vi "FisHRateZ-Main.vi"() -> ()   [LabVIEW 2014]
uses:
  ND2_Reader_32bit/controls/cluster_LIMLOCALMETADATA.ctl
  QSM/Queue_TESTGUIUPDATE/Controls/TypeDef_FrontPanelReferences.ctl
  QSM/Queue_TEST/Controls/QSM_RunStates.ctl
  QSM/Queue_TESTGUIUPDATE/Controls/QSM_RunStates.ctl
  Custom Controls/cluster - Image Results.ctl
  Utilities/Global - Demo Mode Flags.vi
  ND2_Reader_32bit/ND2_Reader_32.lvlib
  QSM/Queue_TESTGUIUPDATE/GUIUpdateQSM.lvlib
  QSM/QueueMaintenance/QueueMaintenance.lvlib
  QSM/Queue_TEST/TestQSM.lvlib
panel:
  in  "About":bool
  in  "Show ROI Detection GUI":bool
  in  "Directory ROI Processing":bool
  in  "Directory Complete Processing":bool
  in  "System Parameters":bool
  in  "Single ROI Calc":bool
  in  "Single File Processing":bool
  in  "Exit":bool
  out "ROI Found?":bool
  in  "Stop Processing":bool
  out "Status":string
  in  "Tab Control":T1(tab)
  in  "Original Image Zoom to Fit":bool
  in  "ROI FOUND Zoom to Fit":bool
  out "LIMLOCALMETADATA":T2 {"dTimeMSec" format="%.2f"}
  out "ROIS":dbl[](array[numeric]) format="%#.2g"
  out "Original Image":T3(plugin-control)
  out "ROI Found":T3(plugin-control)
  out "File":string
  out "XY Graph":cluster{"X":dbl[], "Y":dbl[]}[](graph)
  out "Results String":string
  out "Image Copy":T3(plugin-control)
  in  "Copy Zoom to Fit Image":bool
  in  "Save ROI Results":bool
  out "ROI Results":T4(array[cluster]) {"ROI Values" format="%#.2g"}
  # "* Note: Processing will go faster if 'Original Image' Tab is hidden"
  # "File"
  # "ROI FOUND?"
  # "ROI Values of First Frame"
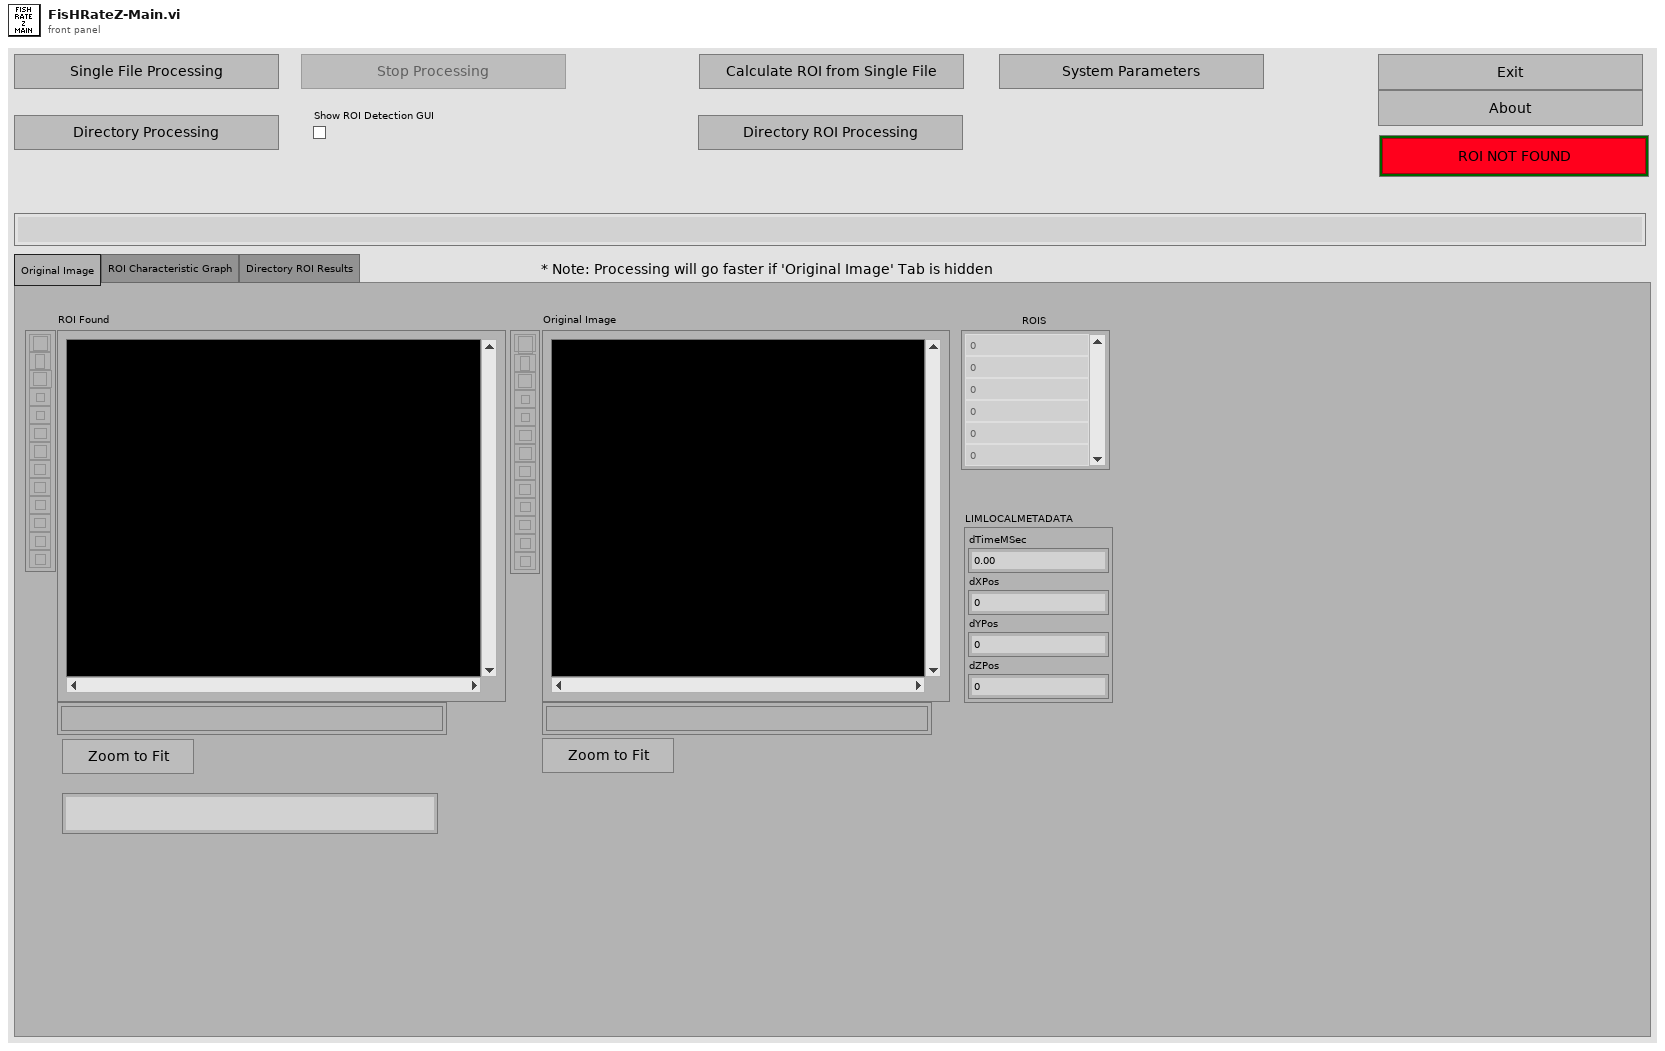
[diagram p1: front panel]
types:
  T1 = enum32{"Original Image", "ROI Characteristic Graph", "Directory ROI Results"}
  T2 = typedef "cluster_LIMLOCALMETADATA.ctl" = cluster{"dTimeMSec":dbl, "dXPos":dbl, "dYPos":dbl, "dZPos":dbl}
  T3 = typedef "IMAQ Image.ctl" = refnum<image>
  T4 = cluster{"File":string, "ROI Found?":bool, "ROI Values":dbl[]}[]
  T5 = typedef "GUIUpdateQSM.lvlib/TypeDef_FrontPanelReferences.ctl" = cluster{"Start":refnum<vi>, "Stop":refnum<vi>, "Status":refnum<vi>, "Exit Button":refnum<vi>, "This VI":refnum<vi>, "System Parameters":refnum<vi>, "Single ROI Calc":refnum<vi>, "ROI X-Y Graph":refnum<vi>, "Directory Complete Processing":refnum<vi>, "Directory ROI Processing":refnum<vi>}
  T6 = typedef "QueueMaintenance.lvlib/QSMRef_ALL.ctl" = cluster{"QSMRef_UpdateUI":T7, "QSMRef_TEST":T8}
  T7 = typedef "GUIUpdateQSM.lvlib/QSM_Reference.ctl" = refnum<queue>
  T8 = typedef "TestQSM.lvlib/QSM_Reference.ctl" = refnum<queue>
  T9 = typedef "TestQSM.lvlib/QSM_ShiftRegister.ctl" = cluster{"Queue References":T6, "user event in":refnum<user-event>, "Single File to Process":path, "Single Image Results":T10, "Analysis Start":timestamp, "Directory to Process":path, "Index":i32, "All Files to Process":path[], "ROI Process":cluster{"Any ROI FOUND?":bool, "ROIS":T11[], "ROIS Found?":bool[], "Particle Measurements (Pixels)":dbl[][], "Particle Variables":i32[], "N Particles Found":i32, "N ROIS Found":i32, "Circles for each Particle":cluster{"Pos. X":i32, "Pos. Y":i32, "Radius":i32, "Core Area":i32}[]}}
  T10 = typedef "cluster - Image Results.ctl" = cluster{"Filename":path, "ROI Results":cluster{"ROIS":dbl[], "LIMLOCALMETADATA":T2}[], "User Stopped?":bool, "ROI Found?":bool, "Error":errorcluster}
  T11 = typedef "ROI Descriptor" = cluster{"Global Rectangle":i32[], "Contours":cluster{"ID":enum32{"External", "Internal"}, "Type":u32, "Coordinates":i32[]}[]}
  T12 = typedef "TestQSM.lvlib/QSM_RunStates.ctl" = enum16{"NULL", "Sect01-Initialize-00-GROUP.ENQUEUE", "Sect02-Single File_Check for Parameters", "Sect02-Single File_Ask for File", "Sect02-Single File_Run Analysis", "Sect02-Single File_Write Results", "Sect03-Single ROI Calc_Check for Parameters", "Sect03-Single ROI Calc_Ask for File", "Sect03-Single ROI Calc_Run Analysis", "Sect03-Single ROI _Write Results", "Sect12-Full Dir_Check for Parameters", "Sect12-Full Dir_Ask for Dir", "Sect12-Full Dir_Check for Next Image to Process", "Sect12-Full Dir_Run Analysis", "Sect12-Full Dir_Write Results", "Sect12-Full Dir_Check if User Stopped", "Sect13-FullDir ROI Calc_Check for Parameters", "Sect13-FullDir ROI Calc_Ask for Dir", "Sect13-Full Dir ROI Calc_Check for Next Image to Process", "Sect13-Full Dir ROI Calc_Run Analysis", "Sect13-Full Dir ROI Calc_Write Results", "Sect13-Full Dir ROI Calc_Check if User Stopped", "Sect90-GUI_Config_Change UI Before Analysis", "Sect90-GUI_Config_Change UI After Analysis", "Sect90-GUI_Stop Processing Pressed", "Sect90-GUI_Stop Processing Button Set Back to F", "Sect90-GUI_Clear ROIs", "Sect99_EXIT-00-Group.Enqueue", "Sect99_EXIT-01-StopQSM"}
  T13 = cluster{"File":string, "ROI Found? 2":bool, "ROIS 2":dbl[]}[]
  T14 = typedef "GUIUpdateQSM.lvlib/QSM_RunStates.ctl" = enum16{"NULL", "Sect01_Initialize-00_GROUP.ENQUEUE", "Sect01_Initialize-01_SetMainToDefault", "Sect01_Initialize-02_Clear Status Strings", "Sect02_UpdateUI-00_Enable Stop_ Disable Start", "Sect02_UpdateUI-01_Enable Start_Disable Stop", "Sect02_UpdateUI-02_Update Status String", "Sect02_UpdateUI-03_Clear XY-Graph", "Sect03-Open ROI  GUI", "Sect03-Close ROI GUI", "Sect99_EXIT-00_Group.Enqueue", "Sect99_EXIT-01_CloseReferences", "Sect99_EXIT-02_StopQSM"}
  T15 = typedef "cluster_LIMPICTURE.ctl" = cluster{"uiWidth":u32, "uiHeight":u32, "uiBitsPerComp":u32, "uiComponents":u32, "uiWidthBytes":u32, "uiSize":u32, "pImageData":u32}
  T16 = typedef "numeric_LIMFILEHANDLE.ctl" = i32
  T17 = cluster{"ROI Calculation":dbl[], "LIMLOCALMETADATA":T2}
  T18 = cluster{"Global Rectangle":i32[], "Contours":cluster{"Contour Type":u32, "ROI Type":u32, "Points":i32[]}[]}
  T19 = cluster{"name":string, "ROI Found?":bool, "ROIS":dbl[]}
  T20 = cluster{"name":string, "ROI Found?":bool, "ROIS":dbl[]}[]
  T21 = typedef "Image Type" = u32
  T22 = cluster{"ROI Calculation":dbl[], "LIMLOCALMETADATA":T2}[]
  T23 = typedef "GUIUpdateQSM.lvlib/QSM_ShiftRegister.ctl" = cluster{"Queue References":T6, "GUI(i) Refs":T5, "user event in":refnum<user-event>}
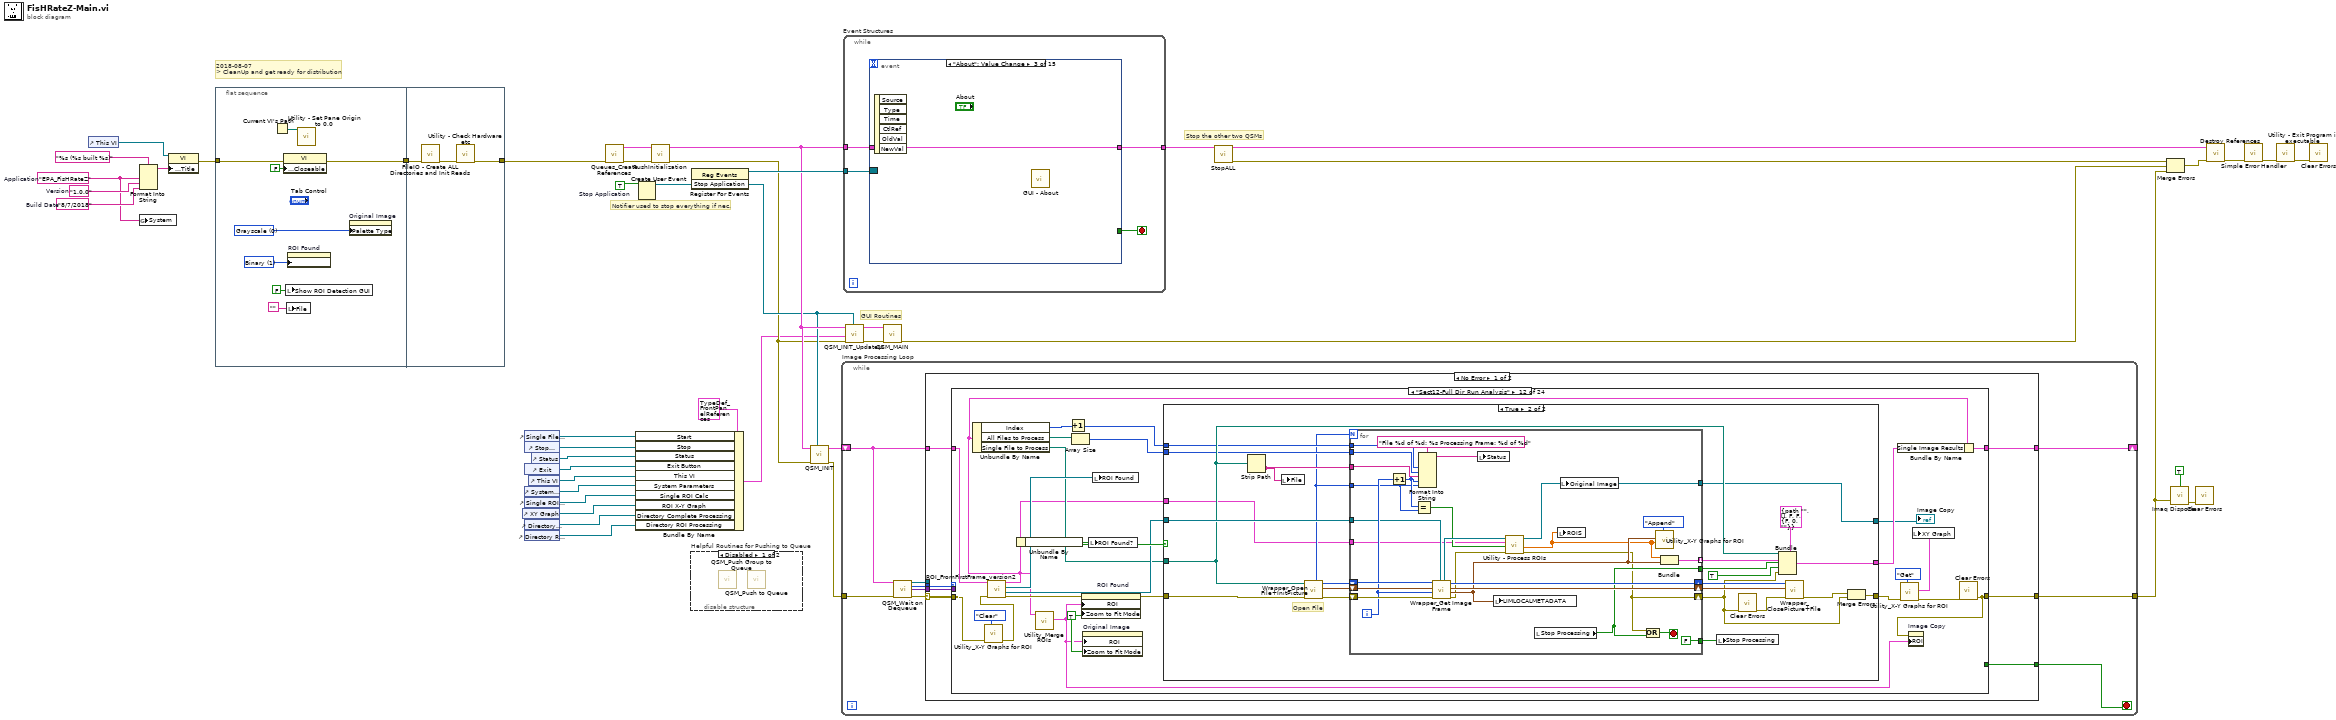
[diagram p0: block diagram]
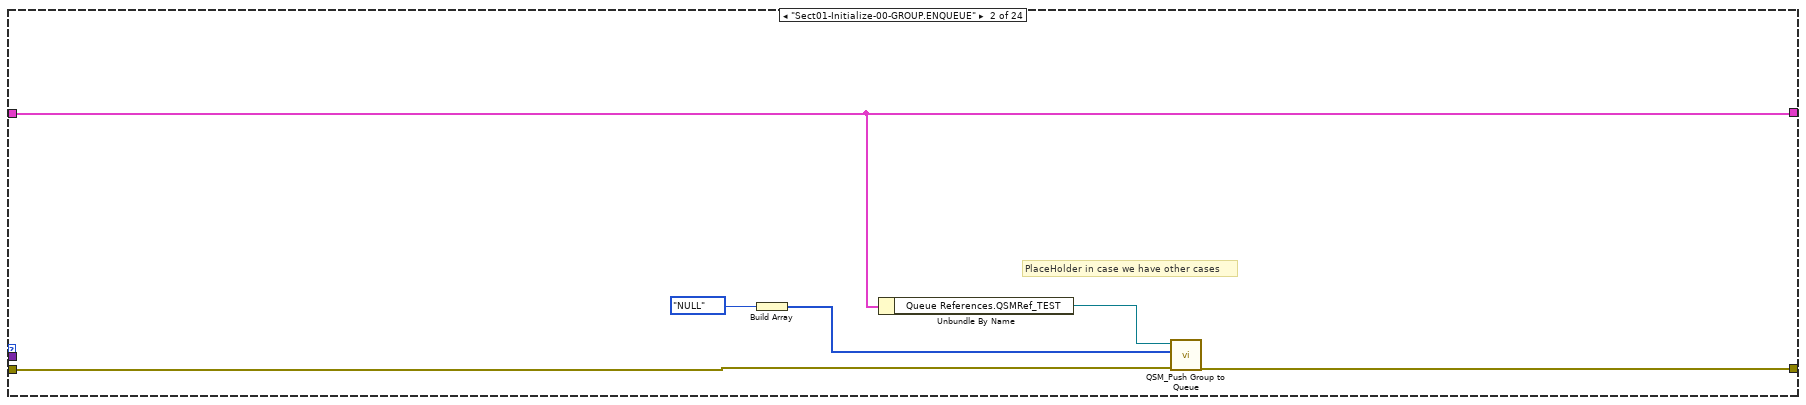
[diagram p4: hidden frame]
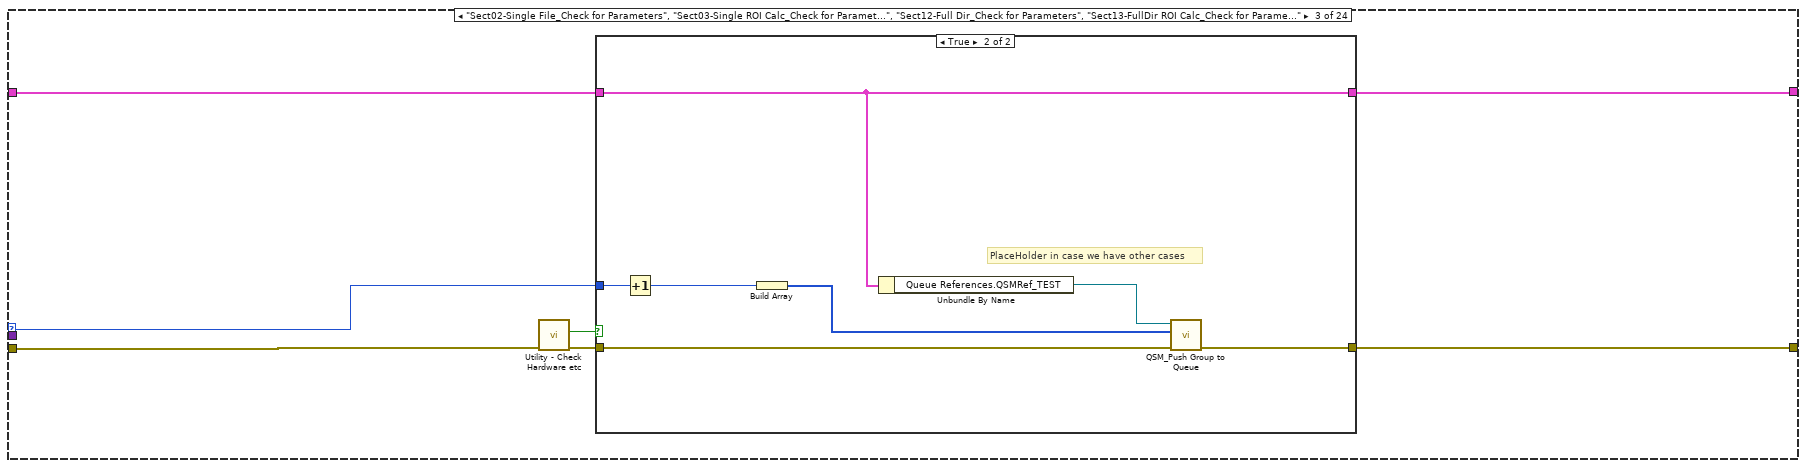
[diagram p5: hidden frame]
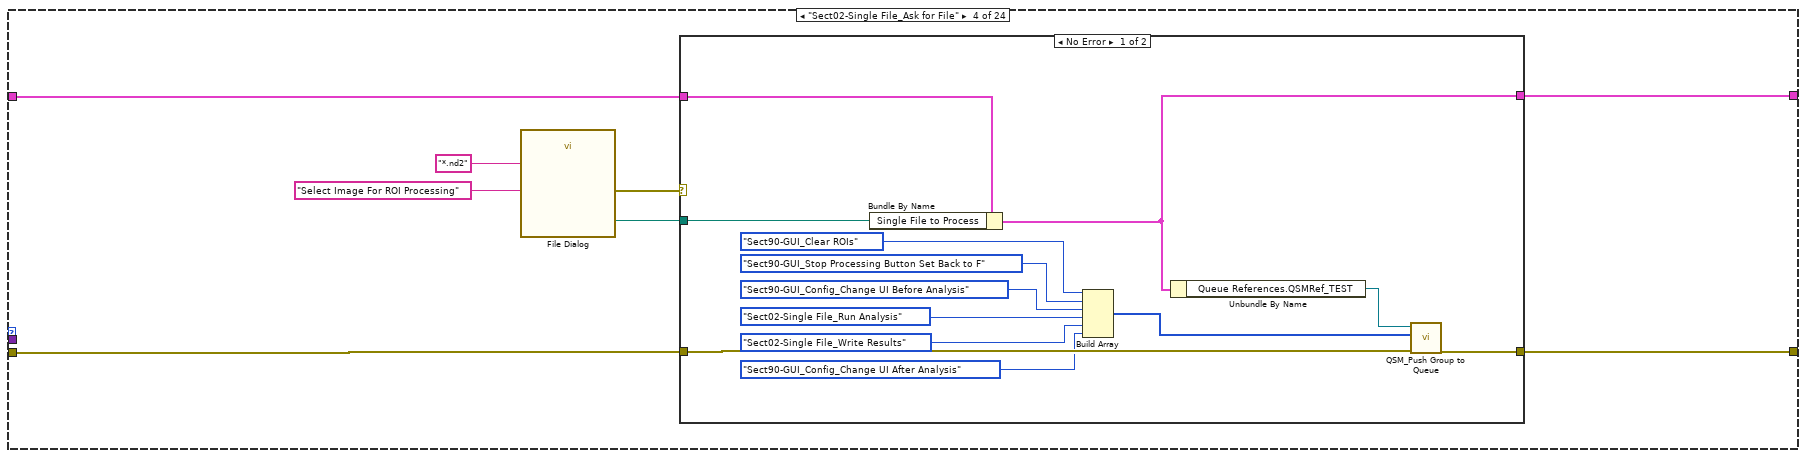
[diagram p7: hidden frame]
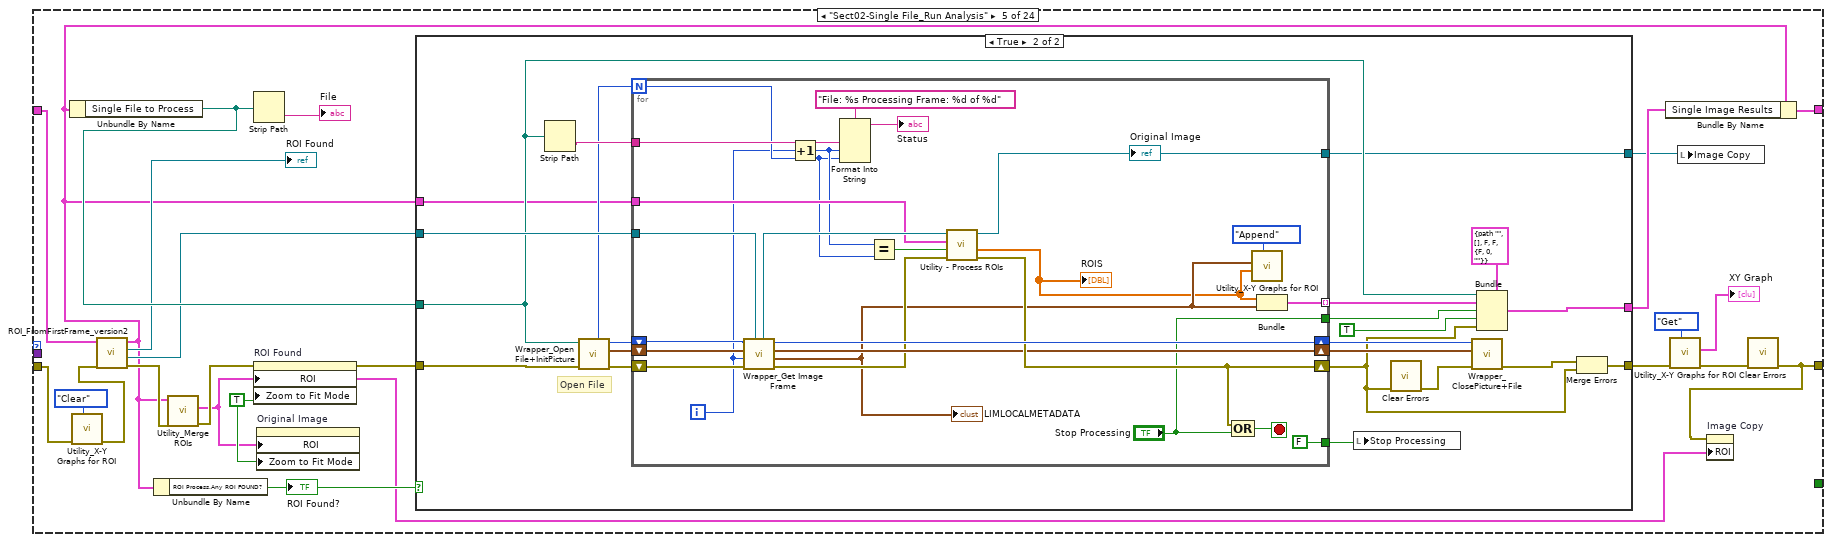
[diagram p9: hidden frame]
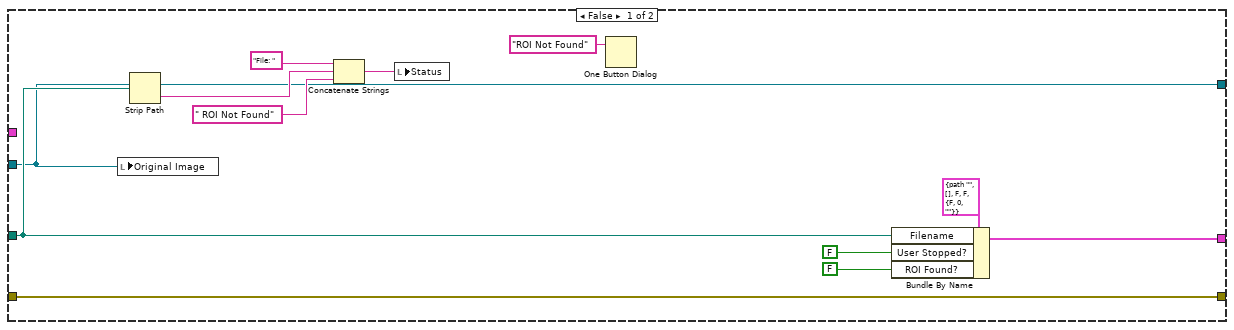
[diagram p10: hidden frame]
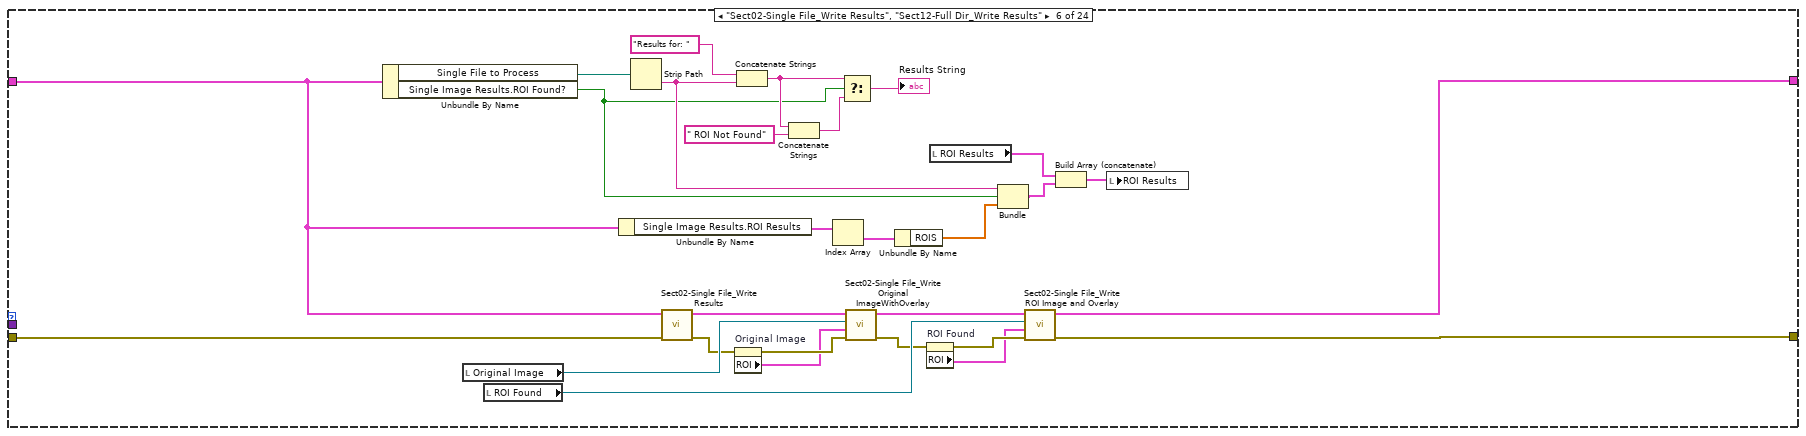
[diagram p11: hidden frame]
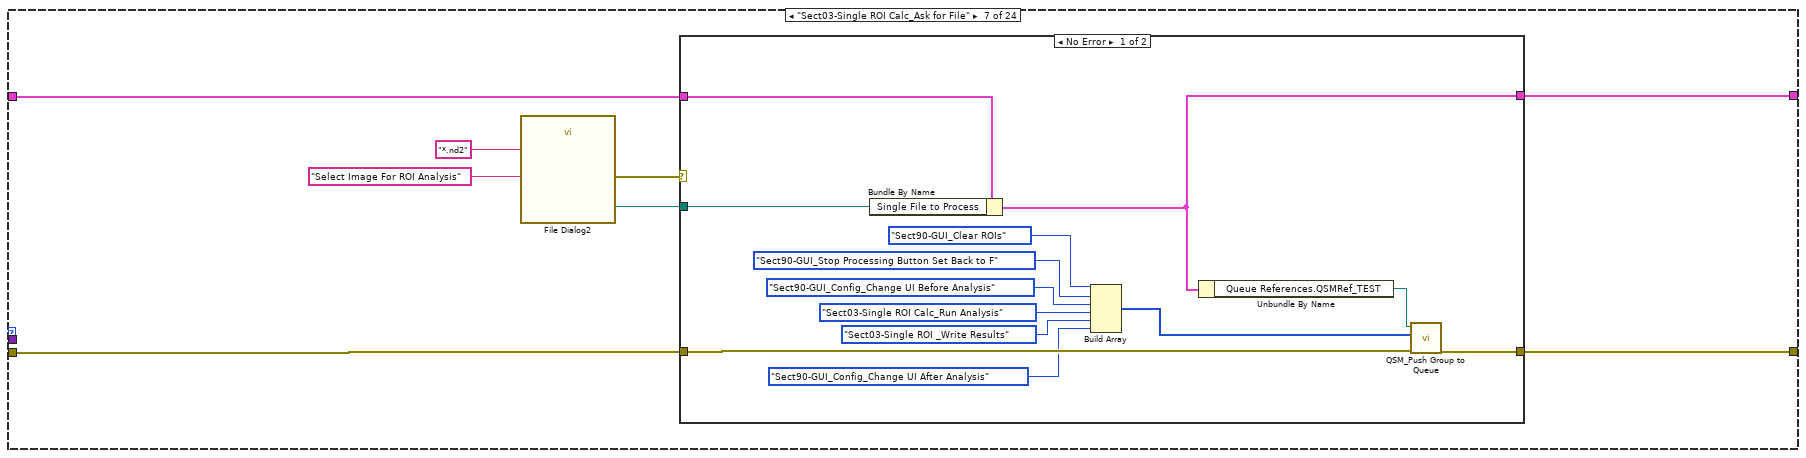
[diagram p12: hidden frame]
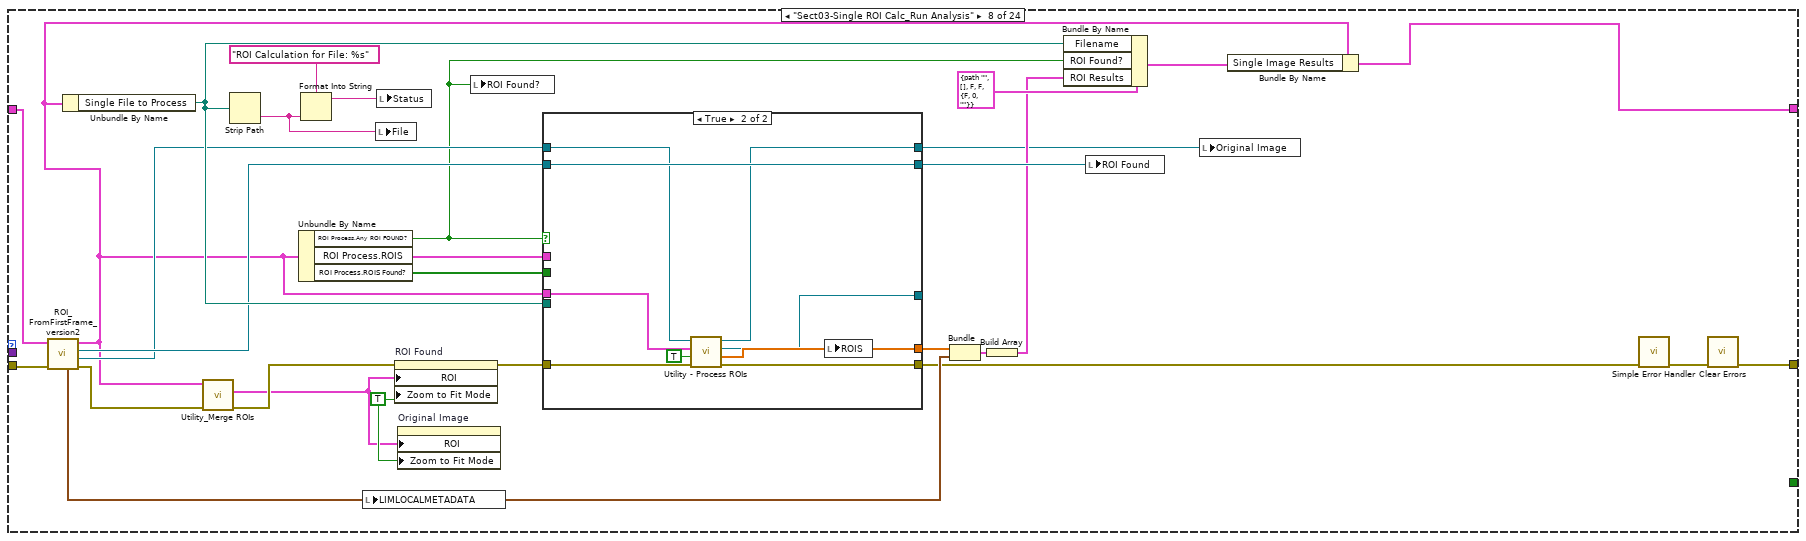
[diagram p14: hidden frame]
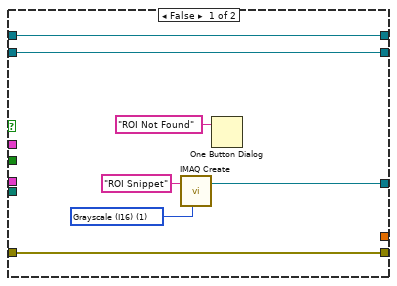
[diagram p15: hidden frame]
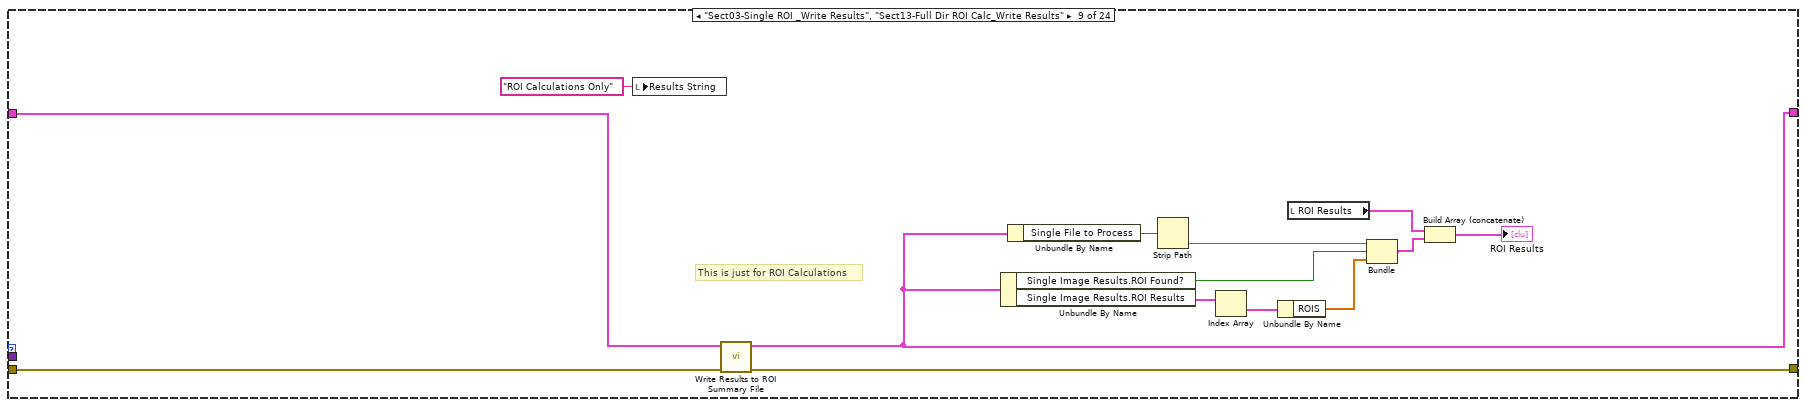
[diagram p16: hidden frame]
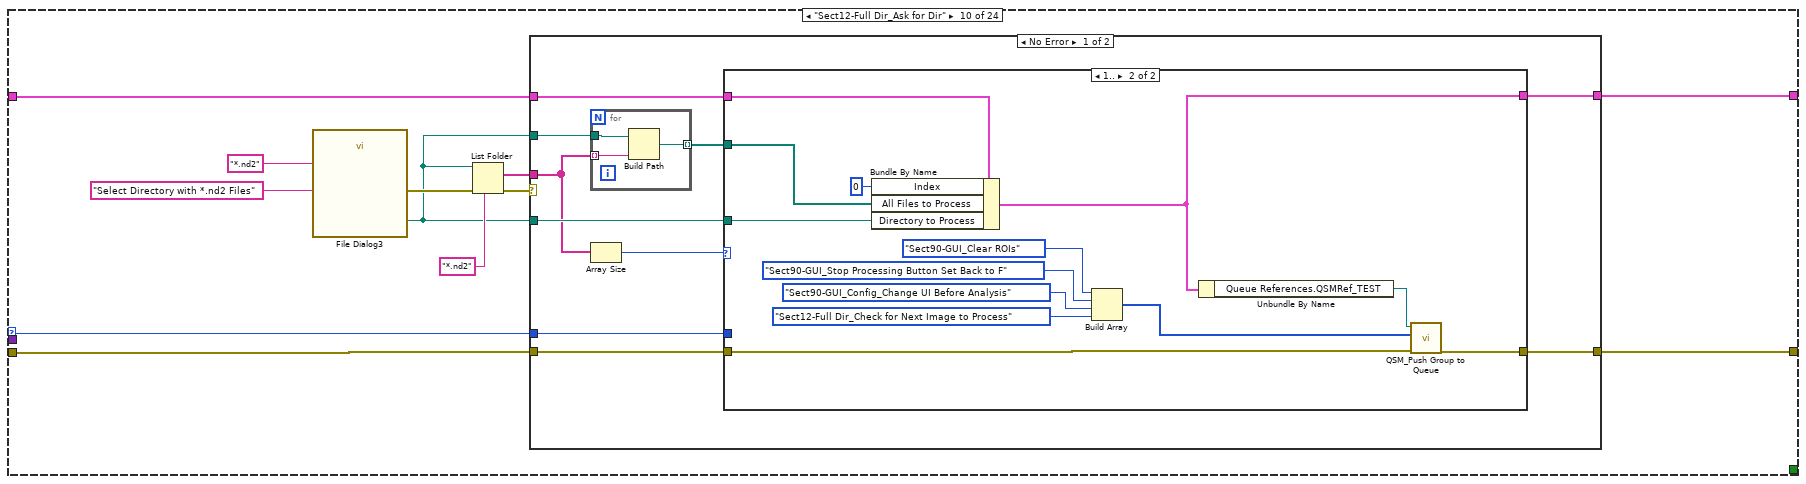
[diagram p17: hidden frame]
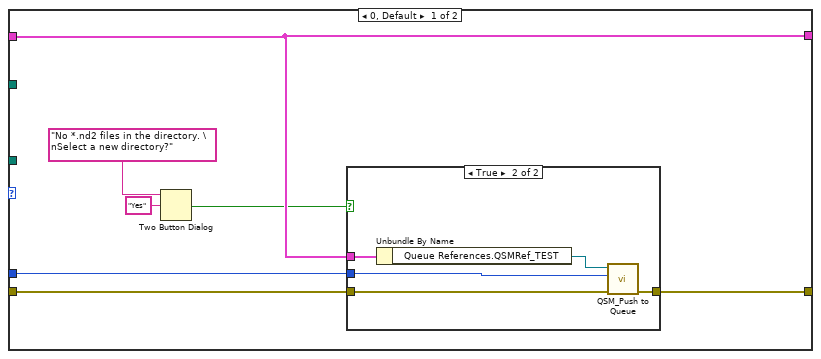
[diagram p18: hidden frame]
diagram:
  w31 = TRUE  # Stop Application
  w42 = "8/7/2018"  # Build Date
  w38 = "EPA_FisHRateZ"  # Application
  w43 = "1.0.0"  # Version
  # "GUI Routines"
  # "Stop the other two QSMs"
  # "2018-08-07\n> CleanUp and get ready for distribution"
  # "Notifier used to stop everything if nec."
  n1 = control-ref of="This VI"() -> (w39:refnum<vi>)
  n2 = Format Into String(format string="%s (%s built %s)", w38, w43, w42) -> (resulting string=w40:string)  [unwired: 2 in, 1 out]
  n3 = global write "Global - Demo Mode Flags.vi" "System"(w38) -> ()
  n4 = property class="VI"(reference=w39, "Front Panel.Title"=w40) -> (error out=w37:errorcluster)  [unwired: 1 in, 1 out]
  n5 = flat-sequence {
    tunnel: w37 -> [w50]
    tunnel: [w46] -> w13
    tunnel: w13 -> [w54]
    tunnel: [w52] -> w12
    frame #0 {
      w49 = u32 1 items=["Grayscale", "Binary", "Gradient", "Rainbow", "Temperature", "User Defined"] ("Palette")
      w48 = u32 0 items=["Grayscale", "Binary", "Gradient", "Rainbow", "Temperature", "User Defined"] ("Palette")
      n6 = Current VI's Path() -> (path=w47:path)
      n7 = property class="VI"(error in=w50, "Front Panel.Closeable"=FALSE ("Front Panel Window:Closeable")) -> (error out=w46:errorcluster)  [unwired: 1 in, 1 out]
      n8 = local write "Show ROI Detection GUI"(FALSE ("Show ROI Detection GUI")) -> ()
      n9 = local write "File"("") -> ()
      n10 = property on="ROI Found" class="ImageControl"("Palette:Palette Type"=w49) -> ()  [unwired: 2 in, 2 out]
      n11 = call "Utility - Set Pane Origin to 0,0.vi"("vi path"=w47) -> ()  [unwired: 10 in, 1 out]
      n12 = property on="Original Image" class="ImageControl"("Palette Type"=w48) -> ()  [unwired: 2 in, 2 out]
    }
    frame #1 {
      n13 = call "FileIO - Create ALL Directories and Init Reads.vi"("error in"=w54) -> ("error out"=w53:errorcluster)  [unwired: 9 in]
      n14 = call "Utility - Check Hardware etc.vi"("error in"=w53) -> ("error out"=w52:errorcluster)  [unwired: 8 in, 1 out]
    }
  }
  n15 = control-ref of="XY Graph"() -> (w8:refnum<vi>)
  n16 = control-ref of="Single File Processing"() -> (w19:refnum<vi>)
  n17 = control-ref of="Stop Processing"() -> (w20:refnum<vi>)
  n18 = control-ref of="Exit"() -> (w17:refnum<vi>)
  n19 = control-ref of="System Parameters"() -> (w15:refnum<vi>)
  n20 = control-ref of="Single ROI Calc"() -> (w9:refnum<vi>)
  n21 = control-ref of="Directory Complete Processing"() -> (w7:refnum<vi>)
  n22 = control-ref of="Directory ROI Processing"() -> (w6:refnum<vi>)
  n23 = control-ref of="This VI"() -> (w16:refnum<vi>)
  n24 = control-ref of="Status"() -> (w18:refnum<vi>)
  n25 = call "Queues_Create References.vi"("error in"=w12) -> ("error out"=w32:errorcluster, "Queue References"=w33:T6)  [unwired: 8 in]
  n26 = Bundle By Name(cluster=T5 {"Start"=refnum, "Stop"=refnum, "Status"=refnum, "Exit Button"=refnum, "This VI"=refnum, "System Parameters"=refnum, "Single ROI Calc"=refnum, "ROI X-Y Graph"=refnum, "Directory Complete Processing"=refnum, "Directory ROI Processing"=refnum} ("FP References"), "Start"=w19, "Stop"=w20, "Status"=w18, "Exit Button"=w17, "This VI"=w16, "System Parameters"=w15, "Single ROI Calc"=w9, "ROI X-Y Graph"=w8, "Directory Complete Processing"=w7, "Directory ROI Processing"=w6) -> (w5:T5)
  n27 = Create User Event(user event datatype=w31) -> (user event=w24:refnum<user-event>)  [unwired: 1 in, 1 out]
  n28 = call "PushInitialization.vi"("error in (no error)"=w32, "Queue References"=w33) -> ("error out"=w10:errorcluster, "Queue References"=w29:T6)  [unwired: 8 in]
  n29 = disable-structure "Helpful Routines for Pushing to Queue" shown="Disabled" {
    frame Disabled {
      n30 = call "QSM_Push Group to Queue.vi"() -> ()  [unwired: 11 in, 1 out]
      n31 = call "QSM_Push to Queue.vi"() -> ()  [unwired: 10 in, 2 out]
    }
    frame Enabled {
    }
  }
  n32 = register-events(w24) -> (reference out=w30:refnum<event-registration>)  [unwired: 2 in, 1 out]
  n33 = call "QSM_INIT.vi"("user event in"=w24, "error in"=w10, "Queue References"=w29) -> ("error out"=w23:errorcluster, "QSM_ShiftRegister_TEST"=w25:T9)  [unwired: 7 in]
  n34 = while "Image Processing Loop" {
    tunnel: [w57] -> w2
    shift-right: [w56] -> _
    shift-left: w25 -> [w63]
    tunnel: w23 -> [w62]
    stop <- w55 stop-if-true
    n35 = call "QSM_Wait on Dequeue.vi"("QSM_ShiftRegister in"=w63, "error in (no error)"=w62) -> ("Queue References.QSMRef out"=w61:T8, "RunStates_TEST"=w59:T12, "DATA.VARIANT"=w58:variant, "error out"=w60:errorcluster)  [unwired: 9 in, 1 out]
    n36 = case shown="No Error" w60 {
      selector: w60 -> [w64 w687]
      tunnel: [w70 w690] -> w57
      tunnel: w63 -> [w67 w689]
      tunnel: w61 -> [_ _]
      tunnel: w59 -> [w69 _]
      tunnel: w58 -> [w68 _]
      tunnel: [w66 w689] -> w56
      tunnel: [w65 TRUE] -> w55
      frame No Error {
        n37 = case shown="\"Sect12-Full Dir_Run Analysis\"" w69 {
          selector: w69 -> [_ _ w79 _ _ _ _ _ _ w310 w371 _ w483 w502 w563 _ w625 _ _ _ _ _ _ _]
          tunnel: w64 -> [w72 w76 w85 w101 w136 w227 w234 w267 w297 w315 w372 w404 w484 w507 w564 w609 w626 w652 w664 w669 w671 w676 w681 w684]
          tunnel: [w72 w75 w84 w100 w118 w216 w233 w277 w296 w320 w374 w392 w486 w512 w566 w604 w628 w651 w656 w665 w671 w676 w680 w684] -> w70
          tunnel: w68 -> [_ _ _ _ _ _ _ _ _ _ _ _ _ _ _ _ _ _ _ _ _ _ _ _]
          tunnel: w67 -> [w71 w78 w82 w102 w130 w200 w235 w262 w298 w321 w370 w400 w482 w513 w562 w588 w624 w655 w663 w668 w672 w677 w683 w686]
          tunnel: [w71 w78 w81 w96 w140 w217 w229 w274 w299 w317 w373 w416 w485 w509 w565 w601 w627 w654 w663 w668 w672 w677 w683 w686] -> w66
          tunnel: [_ _ _ _ _ _ _ _ _ _ _ _ _ _ _ _ _ _ _ _ _ _ _ TRUE] -> w65
          frame "NULL" {
          }
          frame "Sect01-Initialize-00-GROUP.ENQUEUE" {
            # "PlaceHolder in case we have other cases"
            n38 = Build Array(QSM_RunStates."NULL" ("QSM_RunStates_TEST")) -> (w73:T12[])
            n39 = Unbundle By Name(w78) -> ("Queue References.QSMRef_TEST"=w77:T8)
            n40 = call "QSM_Push Group to Queue.vi"("error in (no error)"=w76, "Group Cmds to Push"=w73, "QSM_Reference"=w77) -> ("error out"=w75:errorcluster)  [unwired: 8 in]
          }
          frame "Sect02-Single File_Check for Parameters", "Sect03-Single ROI Calc_Check for Parameters", "Sect12-Full Dir_Check for Parameters", "Sect13-FullDir ROI Calc_Check for Parameters" {
            n41 = call "Utility - Check Hardware etc.vi"("error in"=w85) -> ("error out"=w83:errorcluster, "OK?"=w80:bool)  [unwired: 8 in]
            n42 = case shown="True" w80 {
              tunnel: w82 -> [w87 w90]
              tunnel: [w86 w92] -> w84
              tunnel: w83 -> [w86 w91]
              tunnel: [w87 w90] -> w81
              tunnel: w79 -> [_ w89]
              frame False {
              }
              frame True {
                # "PlaceHolder in case we have other cases"
                n43 = Increment(x=w89) -> (x+1=w88:T12)
                n44 = Build Array(w88) -> (w93:T12[])
                n45 = Unbundle By Name(w90) -> ("Queue References.QSMRef_TEST"=w94:T8)
                n46 = call "QSM_Push Group to Queue.vi"("error in (no error)"=w91, "Group Cmds to Push"=w93, "QSM_Reference"=w94) -> ("error out"=w92:errorcluster)  [unwired: 8 in]
              }
            }
          }
          frame "Sect02-Single File_Ask for File" {
            n47 = call "File Dialog"("prompt"="Select Image For ROI Processing", "pattern (all files)"="*.nd2") -> ("selected path"=w95:path, "error out"=w97:errorcluster)  [unwired: 10 in, 2 out]
            n48 = case shown="No Error" w97 {
              tunnel: w102 -> [w109 w117]
              tunnel: w101 -> [w114 w116]
              tunnel: [w113 w116] -> w100
              tunnel: [w108 w117] -> w96
              tunnel: w95 -> [w110 _]
              frame No Error {
                n49 = Bundle By Name(cluster=w109, "Single File to Process"=w110) -> (w108:T9)
                n50 = Build Array(QSM_RunStates."Sect90-GUI_Clear ROIs" ("QSM_RunStates_TEST"), QSM_RunStates."Sect90-GUI_Stop Processing Button Set Back to F" ("QSM_RunStates_TEST"), QSM_RunStates."Sect90-GUI_Config_Change UI Before Analysis" ("QSM_RunStates_TEST"), QSM_RunStates."Sect02-Single File_Run Analysis" ("QSM_RunStates_TEST"), QSM_RunStates."Sect02-Single File_Write Results" ("QSM_RunStates_TEST"), QSM_RunStates."Sect90-GUI_Config_Change UI After Analysis" ("QSM_RunStates_TEST")) -> (w111:T12[])
                n51 = Unbundle By Name(w108) -> ("Queue References.QSMRef_TEST"=w115:T8)
                n52 = call "QSM_Push Group to Queue.vi"("error in (no error)"=w114, "Group Cmds to Push"=w111, "QSM_Reference"=w115) -> ("error out"=w113:errorcluster)  [unwired: 8 in]
              }
              frame Error {
                # "Cancelled"
              }
            }
          }
          frame "Sect02-Single File_Run Analysis" {
            w134 = TRUE ("Zoom to Fit Mode")
            n53 = call "Utility_X-Y Graphs for ROI.vi"("Graphing Action"=enum16{"Clear", "Append", "Get"}."Clear", "error in (no error)"=w136) -> ("error out"=w135:errorcluster)  [unwired: 8 in, 1 out]
            n54 = call "ROI_FromFirstFrame_version2.vi"("error in"=w135, "QSM_ShiftRegister_TEST in"=w130) -> ("error out"=w127:errorcluster, "Original Image (I16)"=w128:T3, "ROI Out (U8)"=→"ROI Found":T3, "QSM_ShiftRegister_TEST out"=w124:T9)  [unwired: 5 in, 1 out]
            n55 = Unbundle By Name(w124) -> ("Single File to Process"=w131:path)
            n56 = Unbundle By Name(w124) -> ("ROI Process.Any ROI FOUND?"=w125:bool)
            "ROI Found?" <- w125
            n57 = call "Utility_Merge ROIs.vi"("error in (no error)"=w127, "QSM_ShiftRegister_TEST in"=w124) -> ("error out"=w126:errorcluster, "ROI"=w121:T11)  [unwired: 8 in]
            n58 = Strip Path(path=w131) -> (name=→"File":string)  [unwired: 1 out]
            n59 = property on="ROI Found" class="ImageControl"(error in=w126, "ROI"=w121, "Zoom to Fit Mode"=w134) -> (error out=w138:errorcluster)  [unwired: 1 in, 1 out]
            n60 = property on="Original Image" class="ImageControl"("ROI"=w121, "Zoom to Fit Mode"=w134) -> ()  [unwired: 2 in, 2 out]
            n61 = case shown="True" w125 {
              tunnel: w138 -> [w152 w161]
              tunnel: w131 -> [w146 w162]
              tunnel: [w152 w174] -> w122
              tunnel: w128 -> [w141 w171]
              tunnel: [w149 w169] -> w139
              tunnel: w124 -> [_ w154]
              tunnel: [w141 w153] -> w120
              frame False {
                n62 = local write "Original Image"(w141) -> ()
                n63 = Strip Path(path=w146) -> (name=w144:string)  [unwired: 1 out]
                n64 = Concatenate Strings("File: " ("message"), w144, " ROI Not Found" ("message")) -> (w143:string)
                n65 = local write "Status"(w143) -> ()
                n66 = One Button Dialog(message="ROI Not Found") -> ()  [unwired: 1 in, 1 out]
                n67 = Bundle By Name(cluster=T10 {"Filename"=path "", "ROI Results"=[], "User Stopped?"=FALSE, "ROI Found?"=FALSE, "Error"={"status"=FALSE, "code"=0, "source"=""}} ("Single Image Results"), "Filename"=w146, "User Stopped?"=FALSE ("User Stopped? or Error"), "ROI Found?"=FALSE) -> (w149:T10)
              }
              frame True {
                # "Open File"
                n68 = Strip Path(path=w162) -> (name=w173:string)  [unwired: 1 out]
                n69 = call "Wrapper_Open File+InitPicture.vi"("error in (no error)"=w161, "FilePath"=w162) -> ("error out"=w164:errorcluster, "LIMPICTUREout"=w165:T15, "hFile out"=w166:T16, "N Frames (= uiSequenceCount)"=w163:u32)  [unwired: 6 in]
                n70 = for {
                  N: w163 -> [w178]
                  shift-right: [w194] -> w159
                  shift-left: w166 -> [w198]
                  shift-right: [w193] -> w156
                  shift-left: w164 -> [w199]
                  shift-right: [w192] -> w158
                  shift-left: w165 -> [w197]
                  tunnel: w171 -> [w190]
                  tunnel: w173 -> [w189]
                  tunnel: [FALSE ("Stop Processing")] -> w172
                  tunnel: [w187] -> w155 mode=indexing
                  tunnel: ["Stop Processing"] -> w170
                  tunnel: w154 -> [w180]
                  tunnel: [w175] -> w153
                  i -> [w176]
                  stop <- w186 stop-if-true
                  n71 = call "Wrapper_Get Image Frame.vi"("Image Ref in"=w190, "error in (no error)"=w199, "frameindex in"=w176, "LIMPICTURE in"=w197, "hFile in"=w198) -> ("error out"=w191:errorcluster, "LIMLOCALMETADATA"=w183:T2, "LIMPICTURE out"=w192:T15, "hFile out"=w194:T16, "Image Ref out"=w181:T3)  [unwired: 2 in]
                  "LIMLOCALMETADATA" <- w183
                  n72 = Increment(x=w176) -> (x+1=w179:i32)
                  n73 = Format Into String(format string="File: %s Processing Frame: %d of %d", w189, w179, w178) -> (resulting string=→"Status":string)  [unwired: 2 in, 1 out]
                  n74 = Equal?(x=w179, y=w178) -> (x = y?=w177:bool)
                  n75 = call "Utility - Process ROIs.vi"("error in (no error)"=w191, "Overlay?"=w177, "QSM_ShiftRegister_TEST in"=w180, "Original Image In"=w181) -> ("error out"=w193:errorcluster, "ROI Calculation"=w182:dbl[], "Original Image with overlays out"=w175:T3)  [unwired: 4 in, 1 out]
                  "Original Image" <- w175
                  "ROIS" <- w182
                  n76 = Compound Arithmetic op=OR(w193, "Stop Processing") -> (w186:bool)
                  n77 = call "Utility_X-Y Graphs for ROI.vi"("Graphing Action"=enum16{"Clear", "Append", "Get"}."Append", "Data"=w182, "LIMLOCALMETADATA"=w183) -> ()  [unwired: 7 in, 2 out]
                  n78 = Bundle("ROI Calculation"=w182, "LIMLOCALMETADATA"=w183) -> (w187:T17)  [unwired: 1 in]
                }
                n79 = local write "Stop Processing"(w172) -> ()
                n80 = call <vilib>:"Clear Errors.vi"("error in (no error)"=w156) -> ("error out"=w160:errorcluster)  [unwired: 5 in, 1 out]
                n81 = call "Wrapper_ClosePicture+File.vi"("error in (no error)"=w160, "LIMPICTURE"=w158, "hFile in"=w159) -> ("error out"=w157:errorcluster)  [unwired: 8 in]
                n82 = Bundle(cluster=T10 {"Filename"=path "", "ROI Results"=[], "User Stopped?"=FALSE, "ROI Found?"=FALSE, "Error"={"status"=FALSE, "code"=0, "source"=""}} ("Single Image Results"), "Filename"=w162, "ROI Results"=w155, "User Stopped?"=w170, "ROI Found?"=TRUE, "Error"=w156) -> (w169:T10)
                n83 = Merge Errors(w157, w156) -> (w174:errorcluster)
              }
            }
            n84 = Bundle By Name(cluster=w124, "Single Image Results"=w139) -> (w140:T9)
            n85 = call "Utility_X-Y Graphs for ROI.vi"("Graphing Action"=enum16{"Clear", "Append", "Get"}."Get", "error in (no error)"=w122) -> ("error out"=w119:errorcluster, "Graph Out"=→"XY Graph":cluster{"X":dbl[], "Y":dbl[]}[])  [unwired: 8 in]
            n86 = local write "Image Copy"(w120) -> ()
            n87 = call <vilib>:"Clear Errors.vi"("error in (no error)"=w119) -> ("error out"=w118:errorcluster)  [unwired: 5 in, 1 out]
            n88 = property on="Image Copy" class="ImageControl"(error in=w118, "ROI"=w121) -> ()  [unwired: 1 in, 2 out]
          }
          frame "Sect02-Single File_Write Results", "Sect12-Full Dir_Write Results" {
            n89 = Unbundle By Name(w200) -> ("Single File to Process"=w225:path, "Single Image Results.ROI Found?"=w201:bool)
            n90 = local read "Original Image"() -> (w219:T3)
            n91 = local read "ROI Found"() -> (w215:T3)
            n92 = Unbundle By Name(w200) -> ("Single Image Results.ROI Results"=w207:cluster{"ROIS":dbl[], "LIMLOCALMETADATA":T2}[])
            n93 = Strip Path(path=w225) -> (name=w202:string)  [unwired: 1 out]
            n94 = call "Sect02-Single File_Write Results.vi"("error in (no error)"=w227, "QSM_ShiftRegister_TEST in"=w200) -> ("error out"=w214:errorcluster, "QSM_ShiftRegister_TEST out"=w220:T9)  [unwired: 8 in]
            n95 = property on="Original Image" class="ImageControl"(error in=w214) -> (error out=w213:errorcluster, "ROI"=w212:T18)  [unwired: 1 in, 1 out]
            n96 = Concatenate Strings("Results for: " ("string"), w202) -> (w223:string)
            n97 = Concatenate Strings(w223, " ROI Not Found" ("string")) -> (w221:string)
            n98 = Index Array(array=w207) -> (element=w206:cluster{"ROIS":dbl[], "LIMLOCALMETADATA":T2})  [unwired: 1 in]
            n99 = Select(t=w223, s=w201, f=w221) -> (s? t:f=→"Results String":string)
            n100 = call "Sect02-Single File_Write Original ImageWithOverlay.vi"("error in (no error)"=w213, "ROI"=w212, "Original Image (with overlay)"=w219, "QSM_ShiftRegister_TEST in"=w220) -> ("error out"=w211:errorcluster, "QSM_ShiftRegister_TEST out"=w218:T9)  [unwired: 6 in]
            n101 = Unbundle By Name(w206) -> ("ROIS"=w205:dbl[])
            n102 = property on="ROI Found" class="ImageControl"(error in=w211) -> (error out=w210:errorcluster, "ROI"=w209:T18)  [unwired: 1 in, 1 out]
            n103 = local read "ROI Results"() -> (w204:T4)
            n104 = Bundle("name"=w202, "ROI Found?"=w201, "ROIS"=w205) -> (w203:T19)  [unwired: 1 in]
            n105 = call "Sect02-Single File_Write ROI Image and Overlay.vi"("error in (no error)"=w210, "ROI Descriptor"=w209, "ROI Image (with overlay)"=w215, "QSM_ShiftRegister_TEST in"=w218) -> ("error out"=w216:errorcluster, "QSM_ShiftRegister_TEST out"=w217:T9)  [unwired: 6 in]
            n106 = Build Array (concatenate)(w204, w203) -> (w208:T20)
            n107 = local write "ROI Results"(w208) -> ()
          }
          frame "Sect03-Single ROI Calc_Ask for File" {
            n108 = call "File Dialog2"("prompt"="Select Image For ROI Analysis", "pattern (all files)"="*.nd2") -> ("selected path"=w228:path, "error out"=w230:errorcluster)  [unwired: 10 in, 2 out]
            n109 = case shown="No Error" w230 {
              tunnel: w235 -> [w243 w250]
              tunnel: w234 -> [w247 w249]
              tunnel: [w246 w249] -> w233
              tunnel: [w242 w250] -> w229
              tunnel: w228 -> [w244 _]
              frame No Error {
                n110 = Bundle By Name(cluster=w243, "Single File to Process"=w244) -> (w242:T9)
                n111 = Build Array(QSM_RunStates."Sect90-GUI_Clear ROIs" ("QSM_RunStates_TEST"), QSM_RunStates."Sect90-GUI_Stop Processing Button Set Back to F" ("QSM_RunStates_TEST"), QSM_RunStates."Sect90-GUI_Config_Change UI Before Analysis" ("QSM_RunStates_TEST"), QSM_RunStates."Sect03-Single ROI Calc_Run Analysis" ("QSM_RunStates_TEST"), QSM_RunStates."Sect03-Single ROI _Write Results" ("QSM_RunStates_TEST"), QSM_RunStates."Sect90-GUI_Config_Change UI After Analysis" ("QSM_RunStates_TEST")) -> (w245:T12[])
                n112 = Unbundle By Name(w242) -> ("Queue References.QSMRef_TEST"=w248:T8)
                n113 = call "QSM_Push Group to Queue.vi"("error in (no error)"=w247, "Group Cmds to Push"=w245, "QSM_Reference"=w248) -> ("error out"=w246:errorcluster)  [unwired: 8 in]
              }
              frame Error {
                # "Cancelled"
              }
            }
          }
          frame "Sect03-Single ROI Calc_Run Analysis" {
            w264 = TRUE ("Zoom to Fit Mode")
            n114 = call "ROI_FromFirstFrame_version2.vi"("error in"=w267, "QSM_ShiftRegister_TEST in"=w262) -> ("error out"=w259:errorcluster, "Original Image (I16)"=w260:T3, "ROI Out (U8)"=w261:T3, "QSM_ShiftRegister_TEST out"=w254:T9, "LIMLOCALMETADATA"=w269:T2)  [unwired: 5 in]
            n115 = Unbundle By Name(w254) -> ("Single File to Process"=w273:path)
            n116 = call "Utility_Merge ROIs.vi"("error in (no error)"=w259, "QSM_ShiftRegister_TEST in"=w254) -> ("error out"=w258:errorcluster, "ROI"=w252:T11)  [unwired: 8 in]
            n117 = Strip Path(path=w273) -> (name=w263:string)  [unwired: 1 out]
            n118 = Unbundle By Name(w254) -> ("ROI Process.Any ROI FOUND?"=w257:bool, "ROI Process.ROIS"=w256:T11[], "ROI Process.ROIS Found?"=w255:bool[])
            n119 = Format Into String(format string="ROI Calculation for File: %s" ("Status"), w263) -> (resulting string=w276:string)  [unwired: 2 in, 1 out]
            n120 = local write "LIMLOCALMETADATA"(w269) -> ()
            n121 = local write "File"(w263) -> ()
            n122 = local write "Status"(w276) -> ()
            n123 = property on="ROI Found" class="ImageControl"(error in=w258, "ROI"=w252, "Zoom to Fit Mode"=w264) -> (error out=w266:errorcluster)  [unwired: 1 in, 1 out]
            n124 = property on="Original Image" class="ImageControl"("ROI"=w252, "Zoom to Fit Mode"=w264) -> ()  [unwired: 2 in, 2 out]
            n125 = local write "ROI Found?"(w257) -> ()
            n126 = case shown="True" w257 {
              tunnel: w256 -> [_ _]
              tunnel: w266 -> [w285 w294]
              tunnel: w273 -> [_ _]
              tunnel: [w285 w293] -> w251
              tunnel: w260 -> [w283 w292]
              tunnel: [w280 w288] -> _
              tunnel: [w284 w295] -> w279
              tunnel: w261 -> [w284 w295]
              tunnel: [w283 w291] -> w253
              tunnel: [_ w289] -> w270
              tunnel: w255 -> [_ _]
              tunnel: w254 -> [_ w290]
              frame False {
                w282 = T21 1 items=["Grayscale (U8)", "Grayscale (I16)", "Grayscale (SGL)", "Complex (CSG)", "RGB (U32)", "HSL (U32)", "RGB (U64)", "Grayscale (U16)"] ("Image Type")
                n127 = call "IMAQ Create"("Image Name"="ROI Snippet", "Image Type"=w282) -> ("New Image"=w280:T3)  [unwired: 2 in, 2 out]
                n128 = One Button Dialog(message="ROI Not Found") -> ()  [unwired: 1 in, 1 out]
              }
              frame True {
                n129 = call "Utility - Process ROIs.vi"("error in (no error)"=w294, "Overlay?"=TRUE, "QSM_ShiftRegister_TEST in"=w290, "Original Image In"=w292) -> ("error out"=w293:errorcluster, "ROI Calculation"=w289:dbl[], "ROI Snippet Out"=w288:T3, "Original Image with overlays out"=w291:T3)  [unwired: 4 in]
                n130 = local write "ROIS"(w289) -> ()
              }
            }
            n131 = Bundle("ROI Calculation"=w270, "LIMLOCALMETADATA"=w269) -> (w268:T17)  [unwired: 1 in]
            n132 = Build Array(w268) -> (w265:T22)
            n133 = Bundle By Name(cluster=T10 {"Filename"=path "", "ROI Results"=[], "User Stopped?"=FALSE, "ROI Found?"=FALSE, "Error"={"status"=FALSE, "code"=0, "source"=""}} ("Single Image Results"), "Filename"=w273, "ROI Found?"=w257, "ROI Results"=w265) -> (w272:T10)
            n134 = local write "ROI Found"(w279) -> ()
            n135 = local write "Original Image"(w253) -> ()
            n136 = Bundle By Name(cluster=w254, "Single Image Results"=w272) -> (w274:T9)
            n137 = call <vilib>:"Simple Error Handler.vi"("error in (no error)"=w251) -> ("error out"=w278:errorcluster)  [unwired: 4 in, 4 out]
            n138 = call <vilib>:"Clear Errors.vi"("error in (no error)"=w278) -> ("error out"=w277:errorcluster)  [unwired: 5 in, 1 out]
          }
          frame "Sect03-Single ROI _Write Results", "Sect13-Full Dir ROI Calc_Write Results" {
            # "This is just for ROI Calculations"
            n139 = local write "Results String"("ROI Calculations Only" ("Results String")) -> ()
            n140 = call "Write Results to ROI Summary File.vi"("error in (no error)"=w297, "QSM_ShiftRegister_TEST in"=w298) -> ("error out"=w296:errorcluster, "QSM_ShiftRegister_TEST out"=w299:T9)  [unwired: 8 in]
            n141 = Unbundle By Name(w299) -> ("Single Image Results.ROI Found?"=w304:bool, "Single Image Results.ROI Results"=w307:cluster{"ROIS":dbl[], "LIMLOCALMETADATA":T2}[])
            n142 = Unbundle By Name(w299) -> ("Single File to Process"=w308:path)
            n143 = Strip Path(path=w308) -> (name=w305:string)  [unwired: 1 out]
            n144 = Index Array(array=w307) -> (element=w306:cluster{"ROIS":dbl[], "LIMLOCALMETADATA":T2})  [unwired: 1 in]
            n145 = Unbundle By Name(w306) -> ("ROIS"=w303:dbl[])
            n146 = local read "ROI Results"() -> (w302:T4)
            n147 = Bundle("name"=w305, "ROI Found?"=w304, "ROIS"=w303) -> (w300:T19)  [unwired: 1 in]
            n148 = Build Array (concatenate)(w302, w300) -> (→"ROI Results":T20)
          }
          frame "Sect12-Full Dir_Ask for Dir" {
            n149 = call "File Dialog3"("prompt"="Select Directory with *.nd2 Files", "pattern (all files)"="*.nd2") -> ("selected path"=w311:path, "error out"=w314:errorcluster)  [unwired: 10 in, 2 out]
            n150 = List Folder(path=w311, pattern="*.nd2" ("pattern (all files)"), error in=w314) -> (filenames=w312:string[], error out=w313:errorcluster)  [unwired: 1 in, 2 out]
            n151 = case shown="No Error" w313 {
              tunnel: w321 -> [w328 w362]
              tunnel: w315 -> [w331 w361]
              tunnel: [w330 w361] -> w320
              tunnel: [w327 w362] -> w317
              tunnel: w311 -> [w329 _]
              tunnel: w312 -> [w324 _]
              tunnel: w311 -> [w326 _]
              tunnel: w310 -> [w322 _]
              frame No Error {
                n152 = for {
                  tunnel: w326 -> [w360]
                  tunnel: w324 -> [w359] mode=indexing
                  tunnel: [w358] -> w325 mode=indexing
                  n153 = Build Path(base path=w360, name or relative path=w359) -> (appended path=w358:path)
                }
                n154 = Array Size(array=w324) -> (size(s)=w323:i32)
                n155 = case shown="1.." w323 {
                  tunnel: w331 -> [w332 w356]
                  tunnel: [w337 w355] -> w330
                  tunnel: w329 -> [_ w353]
                  tunnel: w328 -> [w336 w352]
                  tunnel: [w336 w351] -> w327
                  tunnel: w325 -> [_ w349]
                  tunnel: w322 -> [w333 _]
                  frame 0, Default {
                    n156 = Two Button Dialog(message="No *.nd2 files in the directory. \nSelect a new directory?", 2:"Yes" ("T button name (\"OK\")")) -> (T button?=w334:bool)  [unwired: 1 in]
                    n157 = case shown="True" w334 {
                      tunnel: [w339 w344] -> w337
                      tunnel: w336 -> [_ w342]
                      tunnel: w333 -> [_ w341]
                      tunnel: w332 -> [w339 w340]
                      frame False {
                      }
                      frame True {
                        n158 = Unbundle By Name(w342) -> ("Queue References.QSMRef_TEST"=w343:T8)
                        n159 = call "QSM_Push to Queue.vi"("error in (no error)"=w340, "QSM_RunStates_TEST"=w341, "QSM_Reference_TEST"=w343) -> ("error out"=w344:errorcluster)  [unwired: 7 in, 1 out]
                      }
                    }
                  }
                  frame 1.. {
                    n160 = Bundle By Name(cluster=w352, "Index"=0, "All Files to Process"=w349, "Directory to Process"=w353) -> (w351:T9)
                    n161 = Build Array(QSM_RunStates."Sect90-GUI_Clear ROIs" ("QSM_RunStates_TEST"), QSM_RunStates."Sect90-GUI_Stop Processing Button Set Back to F" ("QSM_RunStates_TEST"), QSM_RunStates."Sect90-GUI_Config_Change UI Before Analysis" ("QSM_RunStates_TEST"), QSM_RunStates."Sect12-Full Dir_Check for Next Image to Process" ("QSM_RunStates_TEST")) -> (w354:T12[])
                    n162 = Unbundle By Name(w351) -> ("Queue References.QSMRef_TEST"=w357:T8)
                    n163 = call "QSM_Push Group to Queue.vi"("error in (no error)"=w356, "Group Cmds to Push"=w354, "QSM_Reference"=w357) -> ("error out"=w355:errorcluster)  [unwired: 8 in]
                  }
                }
              }
              frame Error {
                # "Cancelled"
              }
            }
          }
          frame "Sect12-Full Dir_Check for Next Image to Process" {
            n164 = Unbundle By Name(w370) -> ("All Files to Process"=w369:path[], "Index"=w367:i32, "All Files to Process"=w364:path[], "Index"=w365:i32)
            n165 = Index Array(array=w364, index=w365) -> (element=w363:path)
            n166 = Array Size(array=w369) -> (size(s)=w368:i32)
            n167 = Greater?(x=w368, y=w367) -> (0:w366:bool)
            n168 = case "Keep Going?" shown="False" w366 {
              tunnel: w370 -> [w378 w385]
              tunnel: w372 -> [w384 w391]
              tunnel: [w383 w390] -> w374
              tunnel: [w377 w385] -> w373
              tunnel: w371 -> [_ _]
              tunnel: w363 -> [w376 _]
              frame True {
                n169 = Bundle By Name(cluster=w378, "Single File to Process"=w376) -> (w377:T9)
                n170 = Build Array(QSM_RunStates."Sect12-Full Dir_Run Analysis" ("QSM_RunStates_TEST"), QSM_RunStates."Sect12-Full Dir_Write Results" ("QSM_RunStates_TEST"), QSM_RunStates."Sect12-Full Dir_Check if User Stopped" ("QSM_RunStates_TEST")) -> (w381:T12[])
                n171 = Unbundle By Name(w377) -> ("Queue References.QSMRef_TEST"=w382:T8)
                n172 = call "QSM_Push Group to Queue.vi"("error in (no error)"=w384, "Group Cmds to Push"=w381, "QSM_Reference"=w382) -> ("error out"=w383:errorcluster)  [unwired: 8 in]
              }
              frame False {
                n173 = Build Array(QSM_RunStates."Sect90-GUI_Config_Change UI After Analysis" ("QSM_RunStates_TEST"), QSM_RunStates."NULL" ("QSM_RunStates_TEST")) -> (w388:T12[])
                n174 = Unbundle By Name(w385) -> ("Queue References.QSMRef_TEST"=w389:T8)
                n175 = call "QSM_Push Group to Queue.vi"("error in (no error)"=w391, "Group Cmds to Push"=w388, "QSM_Reference"=w389) -> ("error out"=w390:errorcluster)  [unwired: 8 in]
              }
            }
          }
          frame "Sect12-Full Dir_Run Analysis" {
            w402 = TRUE ("Zoom to Fit Mode")
            n176 = call "Utility_X-Y Graphs for ROI.vi"("Graphing Action"=enum16{"Clear", "Append", "Get"}."Clear", "error in (no error)"=w404) -> ("error out"=w403:errorcluster)  [unwired: 8 in, 1 out]
            n177 = call "ROI_FromFirstFrame_version2.vi"("error in"=w403, "QSM_ShiftRegister_TEST in"=w400) -> ("error out"=w409:errorcluster, "Original Image (I16)"=w398:T3, "ROI Out (U8)"=w399:T3, "QSM_ShiftRegister_TEST out"=w396:T9)  [unwired: 5 in, 1 out]
            n178 = Unbundle By Name(w396) -> ("Index"=w413:i32, "All Files to Process"=w414:path[], "Single File to Process"=w397:path)
            n179 = Unbundle By Name(w396) -> ("ROI Process.Any ROI FOUND?"=w401:bool)
            n180 = call "Utility_Merge ROIs.vi"("QSM_ShiftRegister_TEST in"=w396) -> ("ROI"=w393:T11)  [unwired: 9 in, 1 out]
            n181 = Increment(x=w413) -> (x+1=w412:i32)
            n182 = Array Size(array=w414) -> (size(s)=w411:i32)
            n183 = property on="ROI Found" class="ImageControl"(error in=w409, "ROI"=w393, "Zoom to Fit Mode"=w402) -> (error out=w410:errorcluster)  [unwired: 1 in, 1 out]
            n184 = property on="Original Image" class="ImageControl"("ROI"=w393, "Zoom to Fit Mode"=w402) -> ()  [unwired: 2 in, 2 out]
            n185 = local write "ROI Found?"(w401) -> ()
            n186 = local write "ROI Found"(w399) -> ()
            n187 = case shown="True" w401 {
              tunnel: w410 -> [w427 w440]
              tunnel: w397 -> [w422 w441]
              tunnel: [w427 w451] -> w394
              tunnel: w398 -> [w417 w449]
              tunnel: [w425 w447] -> w415
              tunnel: w412 -> [_ w434]
              tunnel: w411 -> [_ w433]
              tunnel: w396 -> [_ w429]
              tunnel: [w417 w428] -> w395
              frame False {
                n188 = Strip Path(path=w422) -> (name=w420:string)  [unwired: 1 out]
                n189 = local write "Original Image"(w417) -> ()
                n190 = Concatenate Strings("File: " ("message"), w420, " ROI Not Found" ("message")) -> (w419:string)
                n191 = local write "Status"(w419) -> ()
                n192 = Bundle By Name(cluster=T10 {"Filename"=path "", "ROI Results"=[], "User Stopped?"=FALSE, "ROI Found?"=FALSE, "Error"={"status"=FALSE, "code"=0, "source"=""}} ("Single Image Results"), "Filename"=w422, "User Stopped?"=FALSE ("User Stopped? or Error"), "ROI Found?"=FALSE) -> (w425:T10)
              }
              frame True {
                # "Open File"
                n193 = Strip Path(path=w441) -> (name=w431:string)  [unwired: 1 out]
                n194 = local write "File"(w431) -> ()
                n195 = call "Wrapper_Open File+InitPicture.vi"("error in (no error)"=w440, "FilePath"=w441) -> ("error out"=w442:errorcluster, "LIMPICTUREout"=w443:T15, "hFile out"=w444:T16, "N Frames (= uiSequenceCount)"=w430:u32)  [unwired: 6 in]
                n196 = for {
                  N: w430 -> [_]
                  shift-right: [w473] -> w438
                  shift-left: w444 -> [w477]
                  shift-right: [w458] -> w435
                  shift-left: w442 -> [w478]
                  shift-right: [w472] -> w437
                  shift-left: w443 -> [w476]
                  tunnel: w449 -> [w471]
                  tunnel: w431 -> [w465]
                  tunnel: [FALSE ("Stop Processing")] -> w450
                  tunnel: [w469] -> w432 mode=indexing
                  tunnel: [w466] -> w448
                  tunnel: w430 -> [w459]
                  tunnel: w434 -> [w464]
                  tunnel: w433 -> [w463]
                  tunnel: w429 -> [w453]
                  tunnel: [w452] -> w428
                  i -> [w475]
                  stop <- w468 stop-if-true
                  n197 = Increment(x=w475) -> (x+1=w460:i32)
                  n198 = Equal?(x=w460, y=w459) -> (x = y?=w455:bool)
                  n199 = Format Into String(format string="File %d of %d: %s Processing Frame: %d of %d", w464, w463, w465, w460, w459) -> (resulting string=w467:string)  [unwired: 2 in, 1 out]
                  n200 = call "Wrapper_Get Image Frame.vi"("Image Ref in"=w471, "error in (no error)"=w478, "frameindex in"=w475, "LIMPICTURE in"=w476, "hFile in"=w477) -> ("error out"=w457:errorcluster, "LIMLOCALMETADATA"=w461:T2, "LIMPICTURE out"=w472:T15, "hFile out"=w473:T16, "Image Ref out"=w456:T3)  [unwired: 2 in]
                  n201 = local write "Status"(w467) -> ()
                  n202 = local write "LIMLOCALMETADATA"(w461) -> ()
                  n203 = call "Utility - Process ROIs.vi"("error in (no error)"=w457, "Overlay?"=w455, "QSM_ShiftRegister_TEST in"=w453, "Original Image In"=w456) -> ("error out"=w458:errorcluster, "ROI Calculation"=w454:dbl[], "Original Image with overlays out"=w452:T3)  [unwired: 4 in, 1 out]
                  n204 = local read "Stop Processing"() -> (w466:bool)
                  n205 = local write "ROIS"(w454) -> ()
                  n206 = local write "Original Image"(w452) -> ()
                  n207 = Compound Arithmetic op=OR(w458, w466) -> (w468:bool)
                  n208 = call "Utility_X-Y Graphs for ROI.vi"("Graphing Action"=enum16{"Clear", "Append", "Get"}."Append", "Data"=w454, "LIMLOCALMETADATA"=w461) -> ()  [unwired: 7 in, 2 out]
                  n209 = Bundle("ROI Calculation"=w454, "LIMLOCALMETADATA"=w461) -> (w469:T17)  [unwired: 1 in]
                }
                n210 = local write "Stop Processing"(w450) -> ()
                n211 = call <vilib>:"Clear Errors.vi"("error in (no error)"=w435) -> ("error out"=w439:errorcluster)  [unwired: 5 in, 1 out]
                n212 = Bundle(cluster=T10 {"Filename"=path "", "ROI Results"=[], "User Stopped?"=FALSE, "ROI Found?"=FALSE, "Error"={"status"=FALSE, "code"=0, "source"=""}} ("Single Image Results"), "Filename"=w441, "ROI Results"=w432, "User Stopped?"=w448, "ROI Found?"=TRUE, "Error"=w435) -> (w447:T10)
                n213 = call "Wrapper_ClosePicture+File.vi"("error in (no error)"=w439, "LIMPICTURE"=w437, "hFile in"=w438) -> ("error out"=w436:errorcluster)  [unwired: 8 in]
                n214 = Merge Errors(w436, w435) -> (w451:errorcluster)
              }
            }
            "Image Copy" <- w395
            n215 = Bundle By Name(cluster=w396, "Single Image Results"=w415) -> (w416:T9)
            n216 = call "Utility_X-Y Graphs for ROI.vi"("Graphing Action"=enum16{"Clear", "Append", "Get"}."Get", "error in (no error)"=w394) -> ("error out"=w407:errorcluster, "Graph Out"=w406:cluster{"X":dbl[], "Y":dbl[]}[])  [unwired: 8 in]
            n217 = local write "XY Graph"(w406) -> ()
            n218 = call <vilib>:"Clear Errors.vi"("error in (no error)"=w407) -> ("error out"=w392:errorcluster)  [unwired: 5 in, 1 out]
            n219 = property on="Image Copy" class="ImageControl"(error in=w392, "ROI"=w393) -> ()  [unwired: 1 in, 2 out]
          }
          frame "Sect12-Full Dir_Check if User Stopped" {
            n220 = Unbundle By Name(w482) -> ("Single Image Results.User Stopped?"=w480:bool)
            n221 = local read "Stop Processing"() -> (w479:bool)
            n222 = Compound Arithmetic op=OR(w480, w479) -> (w481:bool)
            n223 = case "User Stopped?" shown="True" w481 {
              tunnel: w482 -> [w488 w493]
              tunnel: w484 -> [w492 w501]
              tunnel: [w491 w500] -> w486
              tunnel: [w488 w494] -> w485
              tunnel: w483 -> [_ _]
              frame True {
                n224 = Unbundle By Name(w488) -> ("Queue References.QSMRef_TEST"=w490:T8)
                n225 = Build Array(QSM_RunStates."Sect90-GUI_Config_Change UI After Analysis" ("QSM_RunStates_TEST")) -> (w489:T12[])
                n226 = call "QSM_Push Group to Queue.vi"("error in (no error)"=w492, "Group Cmds to Push"=w489, "QSM_Reference"=w490) -> ("error out"=w491:errorcluster)  [unwired: 8 in]
              }
              frame False {
                n227 = Unbundle By Name(w493) -> ("Index"=w496:i32)
                n228 = Increment(x=w496) -> (x+1=w495:i32)
                n229 = Bundle By Name(cluster=w493, "Index"=w495) -> (w494:T9)
                n230 = Build Array(QSM_RunStates."Sect12-Full Dir_Check for Next Image to Process" ("QSM_RunStates_TEST")) -> (w498:T12[])
                n231 = Unbundle By Name(w494) -> ("Queue References.QSMRef_TEST"=w499:T8)
                n232 = call "QSM_Push Group to Queue.vi"("error in (no error)"=w501, "Group Cmds to Push"=w498, "QSM_Reference"=w499) -> ("error out"=w500:errorcluster)  [unwired: 8 in]
              }
            }
          }
          frame "Sect13-FullDir ROI Calc_Ask for Dir" {
            n233 = call "File Dialog4"("prompt"="Select Directory with *.nd2 Files", "pattern (all files)"="*.nd2") -> ("selected path"=w503:path, "error out"=w506:errorcluster)  [unwired: 10 in, 2 out]
            n234 = List Folder(path=w503, pattern="*.nd2" ("pattern (all files)"), error in=w506) -> (filenames=w504:string[], error out=w505:errorcluster)  [unwired: 1 in, 2 out]
            n235 = case shown="No Error" w505 {
              tunnel: w513 -> [w520 w554]
              tunnel: w507 -> [w523 w553]
              tunnel: [w522 w553] -> w512
              tunnel: [w519 w554] -> w509
              tunnel: w503 -> [w521 _]
              tunnel: w504 -> [w516 _]
              tunnel: w503 -> [w518 _]
              tunnel: w502 -> [w514 _]
              frame No Error {
                n236 = for {
                  tunnel: w518 -> [w552]
                  tunnel: w516 -> [w551] mode=indexing
                  tunnel: [w550] -> w517 mode=indexing
                  n237 = Build Path(base path=w552, name or relative path=w551) -> (appended path=w550:path)
                }
                n238 = Array Size(array=w516) -> (size(s)=w515:i32)
                n239 = case shown="1.." w515 {
                  tunnel: w523 -> [w524 w548]
                  tunnel: [w529 w547] -> w522
                  tunnel: w521 -> [_ w545]
                  tunnel: w520 -> [w528 w544]
                  tunnel: [w528 w543] -> w519
                  tunnel: w517 -> [_ w541]
                  tunnel: w514 -> [w525 _]
                  frame 0, Default {
                    n240 = Two Button Dialog(message="No *.nd2 files in the directory. \nSelect a new directory?", 2:"Yes" ("T button name (\"OK\")")) -> (T button?=w526:bool)  [unwired: 1 in]
                    n241 = case shown="True" w526 {
                      tunnel: [w531 w536] -> w529
                      tunnel: w528 -> [_ w534]
                      tunnel: w525 -> [_ w533]
                      tunnel: w524 -> [w531 w532]
                      frame False {
                      }
                      frame True {
                        n242 = Unbundle By Name(w534) -> ("Queue References.QSMRef_TEST"=w535:T8)
                        n243 = call "QSM_Push to Queue.vi"("error in (no error)"=w532, "QSM_RunStates_TEST"=w533, "QSM_Reference_TEST"=w535) -> ("error out"=w536:errorcluster)  [unwired: 7 in, 1 out]
                      }
                    }
                  }
                  frame 1.. {
                    n244 = Bundle By Name(cluster=w544, "Index"=0, "All Files to Process"=w541, "Directory to Process"=w545) -> (w543:T9)
                    n245 = Build Array(QSM_RunStates."Sect90-GUI_Clear ROIs" ("QSM_RunStates_TEST"), QSM_RunStates."Sect90-GUI_Stop Processing Button Set Back to F" ("QSM_RunStates_TEST"), QSM_RunStates."Sect90-GUI_Config_Change UI Before Analysis" ("QSM_RunStates_TEST"), QSM_RunStates."Sect13-Full Dir ROI Calc_Check for Next Image to Process" ("QSM_RunStates_TEST")) -> (w546:T12[])
                    n246 = Unbundle By Name(w543) -> ("Queue References.QSMRef_TEST"=w549:T8)
                    n247 = call "QSM_Push Group to Queue.vi"("error in (no error)"=w548, "Group Cmds to Push"=w546, "QSM_Reference"=w549) -> ("error out"=w547:errorcluster)  [unwired: 8 in]
                  }
                }
              }
              frame Error {
                # "Cancelled"
              }
            }
          }
          frame "Sect13-Full Dir ROI Calc_Check for Next Image to Process" {
            n248 = Unbundle By Name(w562) -> ("All Files to Process"=w561:path[], "Index"=w559:i32, "All Files to Process"=w556:path[], "Index"=w557:i32)
            n249 = Index Array(array=w556, index=w557) -> (element=w555:path)
            n250 = Array Size(array=w561) -> (size(s)=w560:i32)
            n251 = Greater?(x=w560, y=w559) -> (0:w558:bool)
            n252 = case "Keep Going?" shown="True" w558 {
              tunnel: w562 -> [w570 w577]
              tunnel: w564 -> [w576 w583]
              tunnel: [w575 w582] -> w566
              tunnel: [w569 w577] -> w565
              tunnel: w563 -> [_ _]
              tunnel: w555 -> [w568 _]
              frame True {
                n253 = Bundle By Name(cluster=w570, "Single File to Process"=w568) -> (w569:T9)
                n254 = Build Array(QSM_RunStates."Sect13-Full Dir ROI Calc_Run Analysis" ("QSM_RunStates_TEST"), QSM_RunStates."Sect13-Full Dir ROI Calc_Write Results" ("QSM_RunStates_TEST"), QSM_RunStates."Sect13-Full Dir ROI Calc_Check if User Stopped" ("QSM_RunStates_TEST")) -> (w573:T12[])
                n255 = Unbundle By Name(w569) -> ("Queue References.QSMRef_TEST"=w574:T8)
                n256 = call "QSM_Push Group to Queue.vi"("error in (no error)"=w576, "Group Cmds to Push"=w573, "QSM_Reference"=w574) -> ("error out"=w575:errorcluster)  [unwired: 8 in]
              }
              frame False {
                n257 = Build Array(QSM_RunStates."Sect90-GUI_Config_Change UI After Analysis" ("QSM_RunStates_TEST"), QSM_RunStates."NULL" ("QSM_RunStates_TEST")) -> (w580:T12[])
                n258 = Unbundle By Name(w577) -> ("Queue References.QSMRef_TEST"=w581:T8)
                n259 = call "QSM_Push Group to Queue.vi"("error in (no error)"=w583, "Group Cmds to Push"=w580, "QSM_Reference"=w581) -> ("error out"=w582:errorcluster)  [unwired: 8 in]
              }
            }
          }
          frame "Sect13-Full Dir ROI Calc_Run Analysis" {
            w590 = TRUE ("Zoom to Fit Mode")
            n260 = call "ROI_FromFirstFrame_version2.vi"("error in"=w609, "QSM_ShiftRegister_TEST in"=w588) -> ("error out"=w593:errorcluster, "Original Image (I16)"=w586:T3, "ROI Out (U8)"=w587:T3, "QSM_ShiftRegister_TEST out"=w584:T9, "LIMLOCALMETADATA"=w595:T2)  [unwired: 5 in]
            n261 = Unbundle By Name(w584) -> ("Single File to Process"=w600:path)
            n262 = Strip Path(path=w600) -> (name=w589:string)  [unwired: 1 out]
            n263 = Format Into String(format string="ROI Calculation for File: %s" ("Status"), w589) -> (resulting string=w603:string)  [unwired: 2 in, 1 out]
            n264 = call "Utility_Merge ROIs.vi"("QSM_ShiftRegister_TEST in"=w584) -> ("ROI"=w591:T11)  [unwired: 9 in, 1 out]
            n265 = Unbundle By Name(w584) -> ("ROI Process.Any ROI FOUND?"=w585:bool)
            n266 = local write "LIMLOCALMETADATA"(w595) -> ()
            n267 = local write "Status"(w603) -> ()
            n268 = local write "File"(w589) -> ()
            n269 = property on="ROI Found" class="ImageControl"(error in=w593, "ROI"=w591, "Zoom to Fit Mode"=w590) -> (error out=w594:errorcluster)  [unwired: 1 in, 1 out]
            n270 = property on="Original Image" class="ImageControl"("ROI"=w591, "Zoom to Fit Mode"=w590) -> ()  [unwired: 2 in, 2 out]
            n271 = local write "ROI Found?"(w585) -> ()
            n272 = case shown="False" w585 {
              tunnel: w594 -> [w612 w619]
              tunnel: [w612 w618] -> w608
              tunnel: w586 -> [w610 w616]
              tunnel: [w611 w620] -> w606
              tunnel: w587 -> [w611 w620]
              tunnel: [w610 w615] -> w607
              tunnel: [_ w617] -> w596
              tunnel: w584 -> [_ w614]
              frame False {
              }
              frame True {
                n273 = call "Utility - Process ROIs.vi"("error in (no error)"=w619, "Overlay?"=TRUE, "QSM_ShiftRegister_TEST in"=w614, "Original Image In"=w616) -> ("error out"=w618:errorcluster, "ROI Calculation"=w617:dbl[], "Original Image with overlays out"=w615:T3)  [unwired: 4 in, 1 out]
                n274 = local write "ROIS"(w617) -> ()
              }
            }
            n275 = Bundle("ROI Calculation"=w596, "LIMLOCALMETADATA"=w595) -> (w597:T17)  [unwired: 1 in]
            n276 = Build Array(w597) -> (w592:T22)
            n277 = Bundle By Name(cluster=T10 {"Filename"=path "", "ROI Results"=[], "User Stopped?"=FALSE, "ROI Found?"=FALSE, "Error"={"status"=FALSE, "code"=0, "source"=""}} ("Single Image Results"), "Filename"=w600, "ROI Found?"=w585, "ROI Results"=w592) -> (w599:T10)
            n278 = local write "Original Image"(w607) -> ()
            n279 = local write "ROI Found"(w606) -> ()
            n280 = Bundle By Name(cluster=w584, "Single Image Results"=w599) -> (w601:T9)
            n281 = call <vilib>:"Simple Error Handler.vi"("error in (no error)"=w608) -> ("error out"=w605:errorcluster)  [unwired: 4 in, 4 out]
            n282 = call <vilib>:"Clear Errors.vi"("error in (no error)"=w605) -> ("error out"=w604:errorcluster)  [unwired: 5 in, 1 out]
          }
          frame "Sect13-Full Dir ROI Calc_Check if User Stopped" {
            n283 = Unbundle By Name(w624) -> ("Single Image Results.User Stopped?"=w622:bool)
            n284 = local read "Stop Processing"() -> (w621:bool)
            n285 = Compound Arithmetic op=OR(w622, w621) -> (w623:bool)
            n286 = case "User Stopped?" shown="False" w623 {
              tunnel: w624 -> [w630 w635]
              tunnel: w626 -> [w634 w643]
              tunnel: [w633 w642] -> w628
              tunnel: [w630 w636] -> w627
              tunnel: w625 -> [_ _]
              frame True {
                n287 = Unbundle By Name(w630) -> ("Queue References.QSMRef_TEST"=w632:T8)
                n288 = Build Array(QSM_RunStates."Sect90-GUI_Config_Change UI After Analysis" ("QSM_RunStates_TEST")) -> (w631:T12[])
                n289 = call "QSM_Push Group to Queue.vi"("error in (no error)"=w634, "Group Cmds to Push"=w631, "QSM_Reference"=w632) -> ("error out"=w633:errorcluster)  [unwired: 8 in]
              }
              frame False {
                n290 = Unbundle By Name(w635) -> ("Index"=w638:i32)
                n291 = Increment(x=w638) -> (x+1=w637:i32)
                n292 = Bundle By Name(cluster=w635, "Index"=w637) -> (w636:T9)
                n293 = Build Array(QSM_RunStates."Sect13-Full Dir ROI Calc_Check for Next Image to Process" ("QSM_RunStates_TEST")) -> (w640:T12[])
                n294 = Unbundle By Name(w636) -> ("Queue References.QSMRef_TEST"=w641:T8)
                n295 = call "QSM_Push Group to Queue.vi"("error in (no error)"=w643, "Group Cmds to Push"=w640, "QSM_Reference"=w641) -> ("error out"=w642:errorcluster)  [unwired: 8 in]
              }
            }
          }
          frame "Sect90-GUI_Config_Change UI Before Analysis" {
            n296 = Build Array(QSM_RunStates."Sect02_UpdateUI-00_Enable Stop_ Disable Start" ("QSM_RunStates_UpdateUI"), QSM_RunStates."Sect02_UpdateUI-03_Clear XY-Graph" ("QSM_RunStates_UpdateUI")) -> (w647:T14[])
            n297 = Unbundle By Name(w655) -> ("Queue References.QSMRef_UpdateUI"=w650:T7)
            n298 = Get Date/Time In Seconds() -> (seconds since 1Jan1904=w653:timestamp)
            n299 = Bundle By Name(cluster=w655, "Analysis Start"=w653) -> (w654:T9)
            n300 = call "QSM_Push Group to Queue.vi"("error in (no error)"=w652, "Group Cmds to Push"=w647, "QSMRef in"=w650) -> ("error out"=w651:errorcluster)  [unwired: 7 in, 1 out]
            n301 = local write "Results String"("") -> ()
            n302 = local write "ROI Results"(T13 [] ("ROI Results")) -> ()
            n303 = property on="ROI Results" class="Arr (strict)"("Index Values"=u32[] [0]) -> ()  [unwired: 2 in, 2 out]
          }
          frame "Sect90-GUI_Config_Change UI After Analysis" {
            n304 = Unbundle By Name(w663) -> ("Queue References.QSMRef_UpdateUI"=w662:T7)
            n305 = call "QSM_Push to Queue.vi"("error in (no error)"=w664, "QSM_RunStates"=QSM_RunStates."Sect02_UpdateUI-01_Enable Start_Disable Stop" ("QSM_RunStates_UpdateUI"), "QSMRef in"=w662) -> ("error out"=w659:errorcluster, "QSMRef out"=w660:T7)  [unwired: 7 in]
            n306 = call "QSM_Push to Queue.vi"("error in (no error)"=w659, "DATA.VARIANT"="Processing Complete", "QSM_RunStates"=QSM_RunStates."Sect02_UpdateUI-02_Update Status String" ("QSM_RunStates_UpdateUI"), "QSMRef in"=w660) -> ("error out"=w656:errorcluster)  [unwired: 6 in, 1 out]
          }
          frame "Sect90-GUI_Stop Processing Pressed" {
            n307 = Unbundle By Name(w668) -> ("Queue References.QSMRef_UpdateUI"=w667:T7)
            n308 = call "QSM_Push to Queue.vi"("error in (no error)"=w669, "QSM_RunStates"=QSM_RunStates."Sect02_UpdateUI-01_Enable Start_Disable Stop" ("QSM_RunStates_UpdateUI"), "QSMRef in"=w667) -> ("error out"=w665:errorcluster)  [unwired: 7 in, 1 out]
          }
          frame "Sect90-GUI_Stop Processing Button Set Back to F" {
            n309 = local write "Stop Processing"(FALSE ("Stop Processing")) -> ()
          }
          frame "Sect90-GUI_Clear ROIs" {
            w674 = T18 {"Global Rectangle"=[], "Contours"=[]} ("ROI")
            w675 = TRUE ("Zoom to Fit Mode")
            n310 = property on="ROI Found" class="ImageControl"("ROI"=w674, "Zoom to Fit Mode"=w675) -> ()  [unwired: 2 in, 2 out]
            n311 = property on="Original Image" class="ImageControl"("ROI"=w674, "Zoom to Fit Mode"=w675) -> ()  [unwired: 2 in, 2 out]
            n312 = local write "ROI Results"(T13 [] ("ROI Results")) -> ()
          }
          frame "Sect99_EXIT-00-Group.Enqueue" {
            # "Placeholder in case we need other actions"
            n313 = Build Array(QSM_RunStates."Sect99_EXIT-01-StopQSM" ("QSM_RunStates_TEST")) -> (w678:T12[])
            n314 = Unbundle By Name(w683) -> ("Queue References.QSMRef_TEST"=w682:T8)
            n315 = call "QSM_Push Group to Queue.vi"("error in (no error)"=w681, "Group Cmds to Push"=w678, "QSM_Reference"=w682) -> ("error out"=w680:errorcluster)  [unwired: 8 in]
          }
          frame "Sect99_EXIT-01-StopQSM" {
          }
        }
      }
      frame Error {
        n316 = call <vilib>:"Clear Errors.vi"("error in (no error)"=w687) -> ("error out"=w690:errorcluster)  [unwired: 5 in, 1 out]
      }
    }
  }
  n317 = while "Event Structures" {
    tunnel: w29 -> [w692]
    tunnel: w30 -> [w693]
    tunnel: [w691] -> w11
    stop <- w694 stop-if-true
    n318 = event shown="[2] \"About\": Value Change" {
      selector: w693 -> [_ _ _ _ _ _ _ _ _ _ _ _ _ _ _]
      dyn-events: _ -> [_ _ _ _ _ _ _ _ _ _ _ _ _ _ _]
      timeout: _ -> [_ _ _ _ _ _ _ _ _ _ _ _ _ _ _]
      tunnel: [_ TRUE _ w700 _ _ _ _ _ _ _ _ _ _ _] -> w694
      tunnel: w692 -> [w695 w696 w698 w699 w703 w709 w711 w715 w717 w721 w724 w727 w729 w731 w733]
      tunnel: [w695 w696 w698 w699 w703 w709 w711 w715 w717 w721 w724 w727 w729 w731 w733] -> w691
      event Timeout {
        n319 = event-data() -> ()  [unwired: 1 in, 2 out]
      }
      event "Exit": Value Change {
        # "Exit and then 'stop all' wil stop the main vi"
        n320 = event-data() -> ()  [unwired: 1 in, 5 out]
      }
      event "About": Value Change {
        n321 = event-data() -> ()  [unwired: 1 in, 6 out]
        n322 = call "GUI - About.vi"() -> ()  [unwired: 12 in]
      }
      event Panel Close? {
        w700 = TRUE ("Discard?")
        n323 = event-data() -> ()  [unwired: 1 in, 3 out]
        n324 = event-data("Discard?"=w700) -> ()  [unwired: 1 in, 1 out]
      }
      event "Single File Processing": Value Change {
        n325 = event-data() -> ()  [unwired: 1 in, 5 out]
        n326 = Unbundle By Name(w703) -> ("QSMRef_TEST"=w702:T8)
        n327 = call "QSM_Push to Queue.vi"("QSM_RunStates_TEST"=QSM_RunStates."Sect02-Single File_Check for Parameters", "QSM_Reference_TEST"=w702) -> ()  [unwired: 8 in, 2 out]
      }
      event "Show ROI Detection GUI": Value Change {
        n328 = event-data() -> ()  [unwired: 1 in, 5 out]
        n329 = Unbundle By Name(w709) -> ("QSMRef_UpdateUI"=w708:T7)
        n330 = Select(t=QSM_RunStates."Sect03-Open ROI  GUI" ("QSM_RunStates_UpdateUI"), s="Show ROI Detection GUI", f=QSM_RunStates."Sect03-Close ROI GUI" ("QSM_RunStates_UpdateUI")) -> (s? t:f=w704:T14)
        n331 = call "QSM_Push to Queue.vi"("QSM_RunStates"=w704, "QSMRef in"=w708) -> ()  [unwired: 8 in, 2 out]
      }
      event "Stop Processing": Value Change {
        n332 = event-data() -> ("NewVal"=w710:bool)  [unwired: 1 in, 4 out]
        n333 = case shown="True" w710 {
          tunnel: w711 -> [_ w714]
          frame False {
          }
          frame True {
            n334 = Unbundle By Name(w714) -> ("QSMRef_TEST"=w713:T8)
            n335 = call "QSM_Push to Queue.vi"("QSM_RunStates_TEST"=QSM_RunStates."Sect90-GUI_Stop Processing Pressed", "QSM_Reference_TEST"=w713) -> ()  [unwired: 8 in, 2 out]
          }
        }
      }
      event "System Parameters": Value Change {
        n336 = event-data() -> ()  [unwired: 1 in, 5 out]
        n337 = Current VI's Path() -> (path=w716:path)
        n338 = call "GUI - System Parameters.vi"("Caller VI FilePath"=w716) -> ()  [unwired: 11 in]
      }
      event "Single ROI Calc": Value Change {
        n339 = event-data() -> ()  [unwired: 1 in, 5 out]
        n340 = Unbundle By Name(w717) -> ("QSMRef_TEST"=w719:T8)
        n341 = call "QSM_Push to Queue.vi"("QSM_RunStates_TEST"=QSM_RunStates."Sect03-Single ROI Calc_Check for Parameters", "QSM_Reference_TEST"=w719) -> ()  [unwired: 8 in, 2 out]
      }
      event "Directory Complete Processing": Value Change {
        n342 = event-data() -> ()  [unwired: 1 in, 5 out]
        n343 = Unbundle By Name(w721) -> ("QSMRef_TEST"=w722:T8)
        n344 = call "QSM_Push to Queue.vi"("QSM_RunStates_TEST"=QSM_RunStates."Sect12-Full Dir_Check for Parameters", "QSM_Reference_TEST"=w722) -> ()  [unwired: 8 in, 2 out]
      }
      event "Directory ROI Processing": Value Change {
        n345 = event-data() -> ()  [unwired: 1 in, 5 out]
        n346 = Unbundle By Name(w724) -> ("QSMRef_TEST"=w725:T8)
        n347 = call "QSM_Push to Queue.vi"("QSM_RunStates_TEST"=QSM_RunStates."Sect13-FullDir ROI Calc_Check for Parameters", "QSM_Reference_TEST"=w725) -> ()  [unwired: 8 in, 2 out]
      }
      event "ROI FOUND Zoom to Fit": Value Change {
        n348 = event-data() -> ()  [unwired: 1 in, 5 out]
        n349 = property on="ROI Found" class="ImageControl"("Zoom to Fit Mode"=TRUE) -> ()  [unwired: 2 in, 2 out]
      }
      event "Original Image Zoom to Fit": Value Change {
        n350 = event-data() -> ()  [unwired: 1 in, 5 out]
        n351 = property on="Original Image" class="ImageControl"("Zoom to Fit Mode"=TRUE) -> ()  [unwired: 2 in, 2 out]
      }
      event "Copy Zoom to Fit Image": Value Change {
        n352 = event-data() -> ()  [unwired: 1 in, 5 out]
        n353 = property on="Image Copy" class="ImageControl"("Zoom to Fit Mode"=TRUE) -> ()  [unwired: 2 in, 2 out]
      }
      event "Save ROI Results": Value Change {
        n354 = event-data() -> ()  [unwired: 1 in, 6 out]
        n355 = local read "ROI Results"() -> (w732:T4)
        n356 = call "FileIO - Save ROI Results.vi"("ROI Results"=w732) -> ()  [unwired: 11 in]
      }
    }
  }
  n357 = call "QSM_INIT_UpdateUI.vi"("user event in"=w24, "error in"=w10, "FP References"=w5, "Queue References"=w29) -> ("error out"=w35:errorcluster, "QSM_ShiftRegister"=w36:T23)  [unwired: 6 in]
  n358 = call "QSM_MAIN.vi"("Error In"=w35, "QSM_ShiftRegister in"=w36) -> ("Error Out"=w26:errorcluster)  [unwired: 8 in, 1 out]
  n359 = call "StopALL.vi"("Queue References In"=w11) -> ("error out"=w28:errorcluster, "Queue ReferencesOut"=w34:T6)  [unwired: 9 in]
  n360 = Merge Errors(w28, w26, w2) -> (w27:errorcluster)
  n361 = call "Imaq Dispose"("All Images? (No)"=TRUE, "error in (no error)"=w2) -> ("error out"=w3:errorcluster)  [unwired: 1 in, 3 out]
  n362 = call <vilib>:"Clear Errors.vi"("error in (no error)"=w3) -> ()  [unwired: 5 in, 2 out]
  n363 = call "Destroy References.vi"("error in"=w27, "Queue References"=w34) -> ("error out"=w22:errorcluster)  [unwired: 8 in]
  n364 = call <vilib>:"Simple Error Handler.vi"("error in (no error)"=w22) -> ("error out"=w21:errorcluster)  [unwired: 4 in, 4 out]
  n365 = call "Utility - Exit Program if executable.vi"("error in (no error)"=w21) -> ("error out"=w14:errorcluster)  [unwired: 10 in]
  n366 = call <vilib>:"Clear Errors.vi"("error in (no error)"=w14) -> ()  [unwired: 5 in, 2 out]
